vi "GyroServoControl In SbRio.vi"() -> ()   [LabVIEW 2017]
uses:
  MsgTypeDef.ctl
  <vilib>/WPC Systems Ltd/GECO Driver/Lib/GECOMotion/GECOMotion/_typedefine/Axis Select.ctl
  <vilib>/WPC Systems Ltd/GECO Driver/Lib/GECOMotion/GECOMotion/GECO Motion.lvclass
  <vilib>/WPC Systems Ltd/GECO Driver/Lib/GECOBase/GECO_Driver Class/Motion/_typedefine/GECO_ActiveHighLow.ctl
  <vilib>/WPC Systems Ltd/GECO Driver/Lib/GECOBase/GECO_Driver Class/GECO_Driver.lvclass
  <vilib>/WPC Systems Ltd/GECO Driver/Lib/GECOBase/GECO_Driver Class/Motion/_typedefine/GECO_Motion Operation Mode.ctl
  <vilib>/addons/control/pid/NI_PID_pid.lvlib
  <vilib>/addons/control/pid/pid.llb/PID (DBL).vi
  <vilib>/WPC Systems Ltd/GECO Driver/GECODriver/GECO_Initialize_PC/Initialize VIs/Initialize_GECOUno_4HX.vi
  <vilib>/NI/Modbus Library/API/Wrapper/API Main.lvlib
  <vilib>/NI/Modbus Library/API/Wrapper/Create TCP Slave.vi
  <vilib>/NI/Modbus Library/API/Modbus API.lvclass
  <vilib>/Instr/_visa.llb/VISA Configure Serial Port (Instr).vi
  GyroDef.ctl
  <vilib>/WPC Systems Ltd/GECO Driver/Lib/GECOBase/GECO_Driver Class/GECO_SlotName.ctl
  <vilib>/WPC Systems Ltd/GECO Driver/Lib/GECOBase/GECO_Driver Class/Motion/_typedefine/GECO_Stepper Output Configuration.ctl
  DataDef.ctl
  <vilib>/NI/Modbus Library/API/Slave/Modbus Slave.lvclass
  C:/Program Files (x86)/National Instruments/LabVIEW 2019/vi.lib/NI/Modbus Library/API/Modbus API.lvclass
  Reverse Polarity.ctl
  Forward Polarity.ctl
  Motion Controller Slot.ctl
  Stepper Output Configuration.ctl
  Axis Select.ctl
panel:
  out "實際角度":cluster{"X":dbl, "Y":dbl}={"X"=-3.299667554384925, "Y"=3.520332445615068}
  out "實際角度Chart":cluster{"X":dbl, "Y":dbl}(graph)={"X"=-3.299667554384925, "Y"=3.520332445615068} caption="Waveform Chart - dark"
  in  "Main Setting Tab":T1(tab)
  in  "TimerON":bool
  in  "Timer(ms)":i32=1
  in  "Serial Port":refnum<visa-resource-name>="COM3"
  in  "TCP slave port":u32=1
  in  "baud rate":u32=115200
  in  "Byte bits":u32=8
  in  "Modbus Address Starting":u32
  in  "Modbus Number of Inputs":u32=10000
  in  "Resource Name":tag="rio://192.168.0.224/RIO0"
  in  "Servo on":bool
  in  "Axis Select":T2
  in  "Stepper Output Configuration":T3=enum."CW/CCW(Two Pulse)"
  in  "Forward Enable?":bool=TRUE
  in  "Reverse Enable?":bool=TRUE
  in  "Motion Operation Mode":T4(ring)=enum."Velocity"
  in  "Forward Polarity":T5
  in  "Reverse Polarity":T6
  in  "Motion Controller Slot":T7
  in  "Target Position (0)":dbl=10000.0
  in  "Acceleration (100000)":u32=300000
  in  "Velocity (10000)":dbl=100000.0
  in  "Deacceleration (100000)":u32=300000
  in  "PID gains setting Tab":enum32{"Axis 1", "Axis 2", "Axis 3"}(tab)
  in  "PID gains":T8={"proportional gain (Kc)"=1.0, "integral time (Ti, min)"=0.01, "derivative time (Td, min)"=0.0} {"derivative time (Td, min)" format="%#_3f"; "integral time (Ti, min)" format="%#_3f"; "proportional gain (Kc)" format="%#_3f"}
  in  "PID gains 2":T8={"proportional gain (Kc)"=1.0, "integral time (Ti, min)"=0.01, "derivative time (Td, min)"=0.0} {"derivative time (Td, min)" format="%#_3f"; "integral time (Ti, min)" format="%#_3f"; "proportional gain (Kc)" format="%#_3f"}
  in  "PID gains 3":T8={"proportional gain (Kc)"=1.0, "integral time (Ti, min)"=0.01, "derivative time (Td, min)"=0.0} {"derivative time (Td, min)" format="%#_3f"; "integral time (Ti, min)" format="%#_3f"; "proportional gain (Kc)" format="%#_3f"}
  in  "ZABStop":bool
  in  "B":i32
  in  "A":i32
  in  "Z":i32=50
  in  "ZAB Start":bool
  in  "Move Setting":T9
  out "register values":dbl[](array[numeric])
  out "Axis 1":T10
  out "Axis 2":T10
  out "Axis 3":T10
  out "cicrle Period":u32
  out "Program Period":u32
  in  "ServoButtonControl":T11
  in  "Connect":bool
  in  "Close":bool
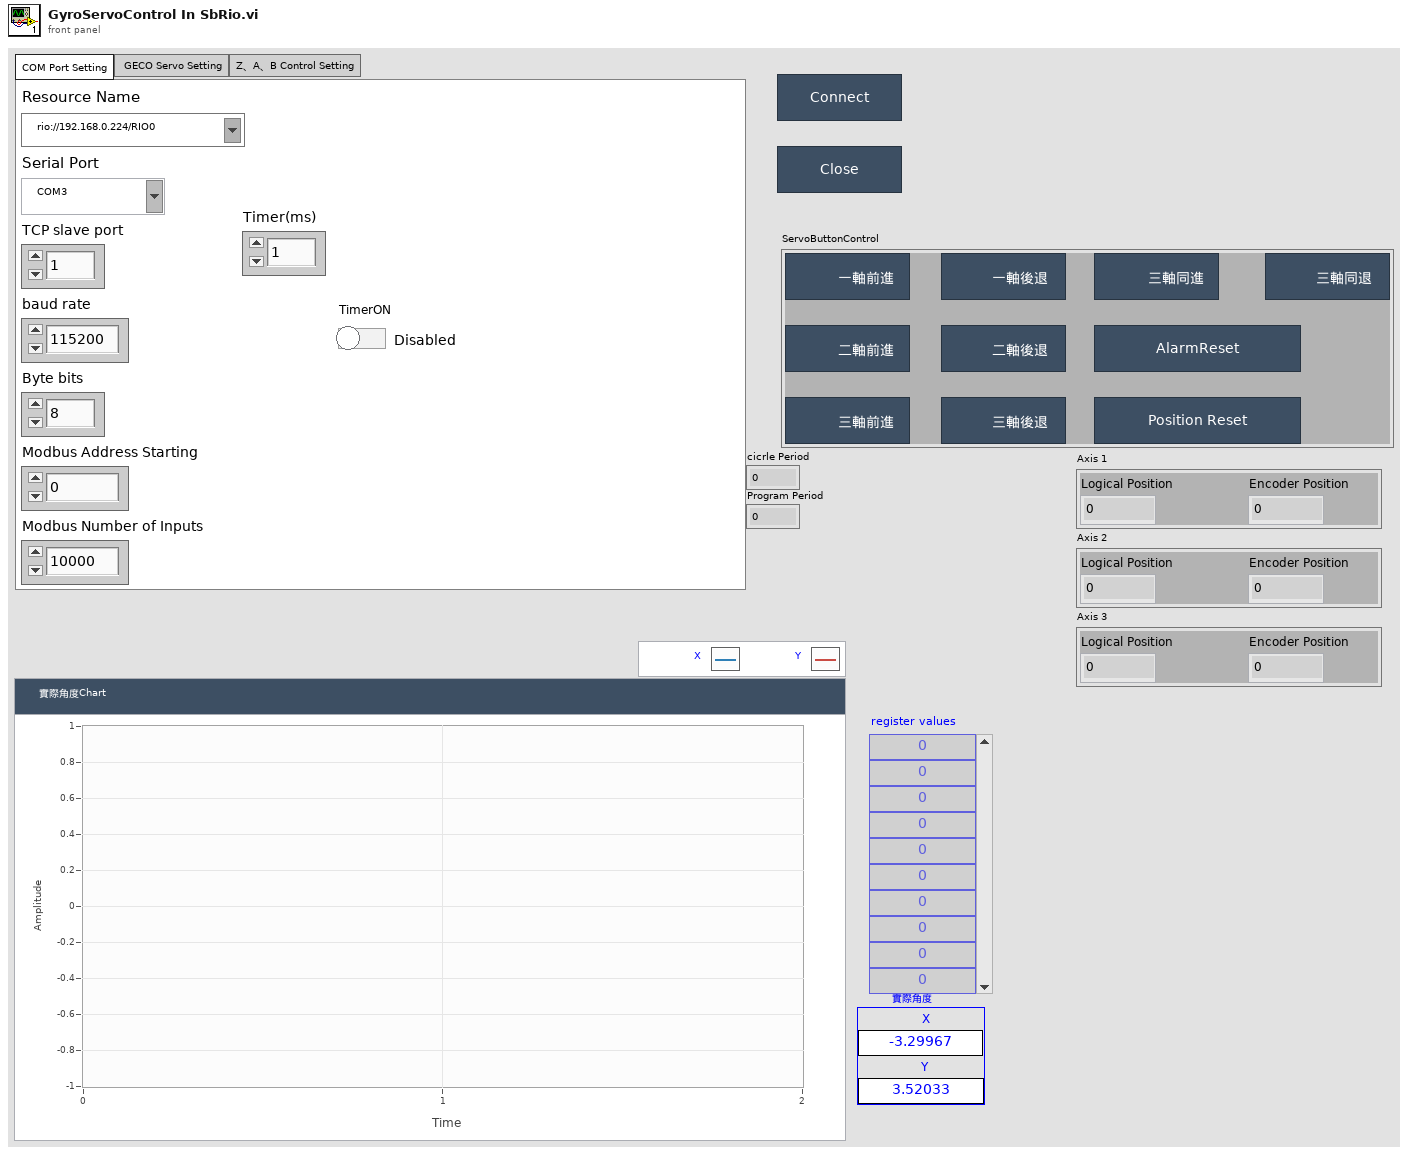
[diagram p1: front panel]
types:
  T1 = enum32{"COM Port Setting", " GECO Servo Setting", "Z、A、B Control Setting"}
  T2 = typedef "Axis Select.ctl" = enum16{"Axis 1", "Axis 2", "Axis 3", "Axis 4"}
  T3 = typedef "Stepper Output Configuration.ctl" = enum16{"Step/Dir(One Pulse)", "CW/CCW(Two Pulse)"}
  T4 = enum16{"Absolute Position", "Relative Position", "Velocity"}
  T5 = typedef "Forward Polarity.ctl" = enum16{"Active High", "Active Low"}
  T6 = typedef "Reverse Polarity.ctl" = enum16{"Active High", "Active Low"}
  T7 = typedef "Motion Controller Slot.ctl" = enum16{"C1", "C2", "C3", "C4"}
  T8 = cluster{"proportional gain (Kc)":dbl, "integral time (Ti, min)":dbl, "derivative time (Td, min)":dbl}
  T9 = typedef "軌跡設定.ctl" = u16
  T10 = cluster{"Encoder Position":i32, "Logical Position":i32}
  T11 = cluster{"三軸同退":bool, "三軸同進":bool, "三軸後退":bool, "三軸前進":bool, "二軸後退":bool, "二軸前進":bool, "一軸後退":bool, "一軸前進":bool, "Reset Encoder Position":bool, "AlarmReset":bool}
  T12 = typedef "DataDef.ctl" = cluster{"address starting":u16, "狀態":enum16{"初始化", "讀取", "寫入", "停止"}, "理想角度":cluster{"A":dbl, "B":dbl}, "register values":i16[], "Modbus COM":refnum<class "Modbus API.lvclass">, "TCP slave port":u16, " baud rate":u32, "Byte bits":u16, "ServoButtonControl":cluster{"三軸同退":bool, "三軸同進":bool, "三軸後退":bool, "三軸前進":bool, "二軸後退":bool, "二軸前進":bool, "一軸後退":bool, "一軸前進":bool}, "Serial Number":string, "GECO_Driver out":refnum<class "GECO_Driver.lvclass">, "number of inputs":u16, "ServoSetting":cluster{"Axis Select":T13, "Stepper Output Configuration":T14, "Motion Operation Mode":T15, "Motion Controller Slot":T16, "Singel Axis Move Paramters":cluster{"Motion Operation Mode":T15, "Target Position (0)":i32, "Velocity (10000)":i32, "Acceleration (100000)":u32, "Deacceleration (100000)":u32}, "Reverse":cluster{"Reverse Enable":bool, "Reverse Polarity":T17}, "Forward":cluster{"Forward Enable":bool, "Forward Polarity":T17}}, "GECO Motion out":refnum<class "GECO Motion.lvclass">, "Servo on":bool, "Axis 1 Position":cluster{"Encoder Position":i32, "Logical Position":i32}, "Axis 2 Position":cluster{"Encoder Position":i32, "Logical Position":i32}, "Axis 3 Position":cluster{"Encoder Position":i32, "Logical Position":i32}, "PIDSetting":cluster{"Z":i32, "A":i32, "B":i32, "Move Setting":T18, "Axis Pulse":dbl, "Axis Length":dbl, "PID gains ":cluster{"proportional gain (Kc)":dbl, "integral time (Ti, min)":dbl, "derivative time (Td, min)":dbl}}, "resource name":tag, "Save Path":refnum<file>}
  T13 = typedef "GECO Motion.lvclass/Axis Select.ctl" = enum16{"Axis 1", "Axis 2", "Axis 3", "Axis 4"}
  T14 = typedef "GECO_Driver.lvclass/GECO_Stepper Output Configuration.ctl" = enum16{"Step/Dir(One Pulse)", "CW/CCW(Two Pulse)"}
  T15 = typedef "GECO_Driver.lvclass/GECO_Motion Operation Mode.ctl" = enum16{"Absolute Position", "Relative Position", "Velocity"}
  T16 = typedef "GECO_Driver.lvclass/GECO_SlotName.ctl" = enum16{"C1", "C2", "C3", "C4"}
  T17 = typedef "GECO_Driver.lvclass/GECO_ActiveHighLow.ctl" = enum16{"Active High", "Active Low"}
  T18 = typedef "­y¸ñ.ctl" = u16
  T19 = typedef "MsgTypeDef.ctl" = cluster{"CMD":string, "DATA":variant}
  T20 = typedef "GyroDef.ctl" = cluster{"Byte bits":u16, "baud rate":u32, "實際角度":cluster{"A":dbl, "B":dbl}, "COM Port":refnum<visa-resource-name>, "Save Path":refnum<file>}
  T21 = cluster{"Motion Operation Mode":T15, "Target Position (0)":i32, "Velocity (10000)":i32, "Acceleration (100000)":u32, "Deacceleration (100000)":u32}
  T22 = cluster{"Forward Enable":bool, "Forward Polarity":T17}
  T23 = cluster{"Reverse Enable":bool, "Reverse Polarity":T17}
  T24 = cluster{"三軸同退":bool, "三軸同進":bool, "三軸後退":bool, "三軸前進":bool, "二軸後退":bool, "二軸前進":bool, "一軸後退":bool, "一軸前進":bool, "Reset Encoder Position":bool, "AlarmReset":bool}[]
  T25 = cluster{"Logical Position":i32, "Encoder Position":i32}
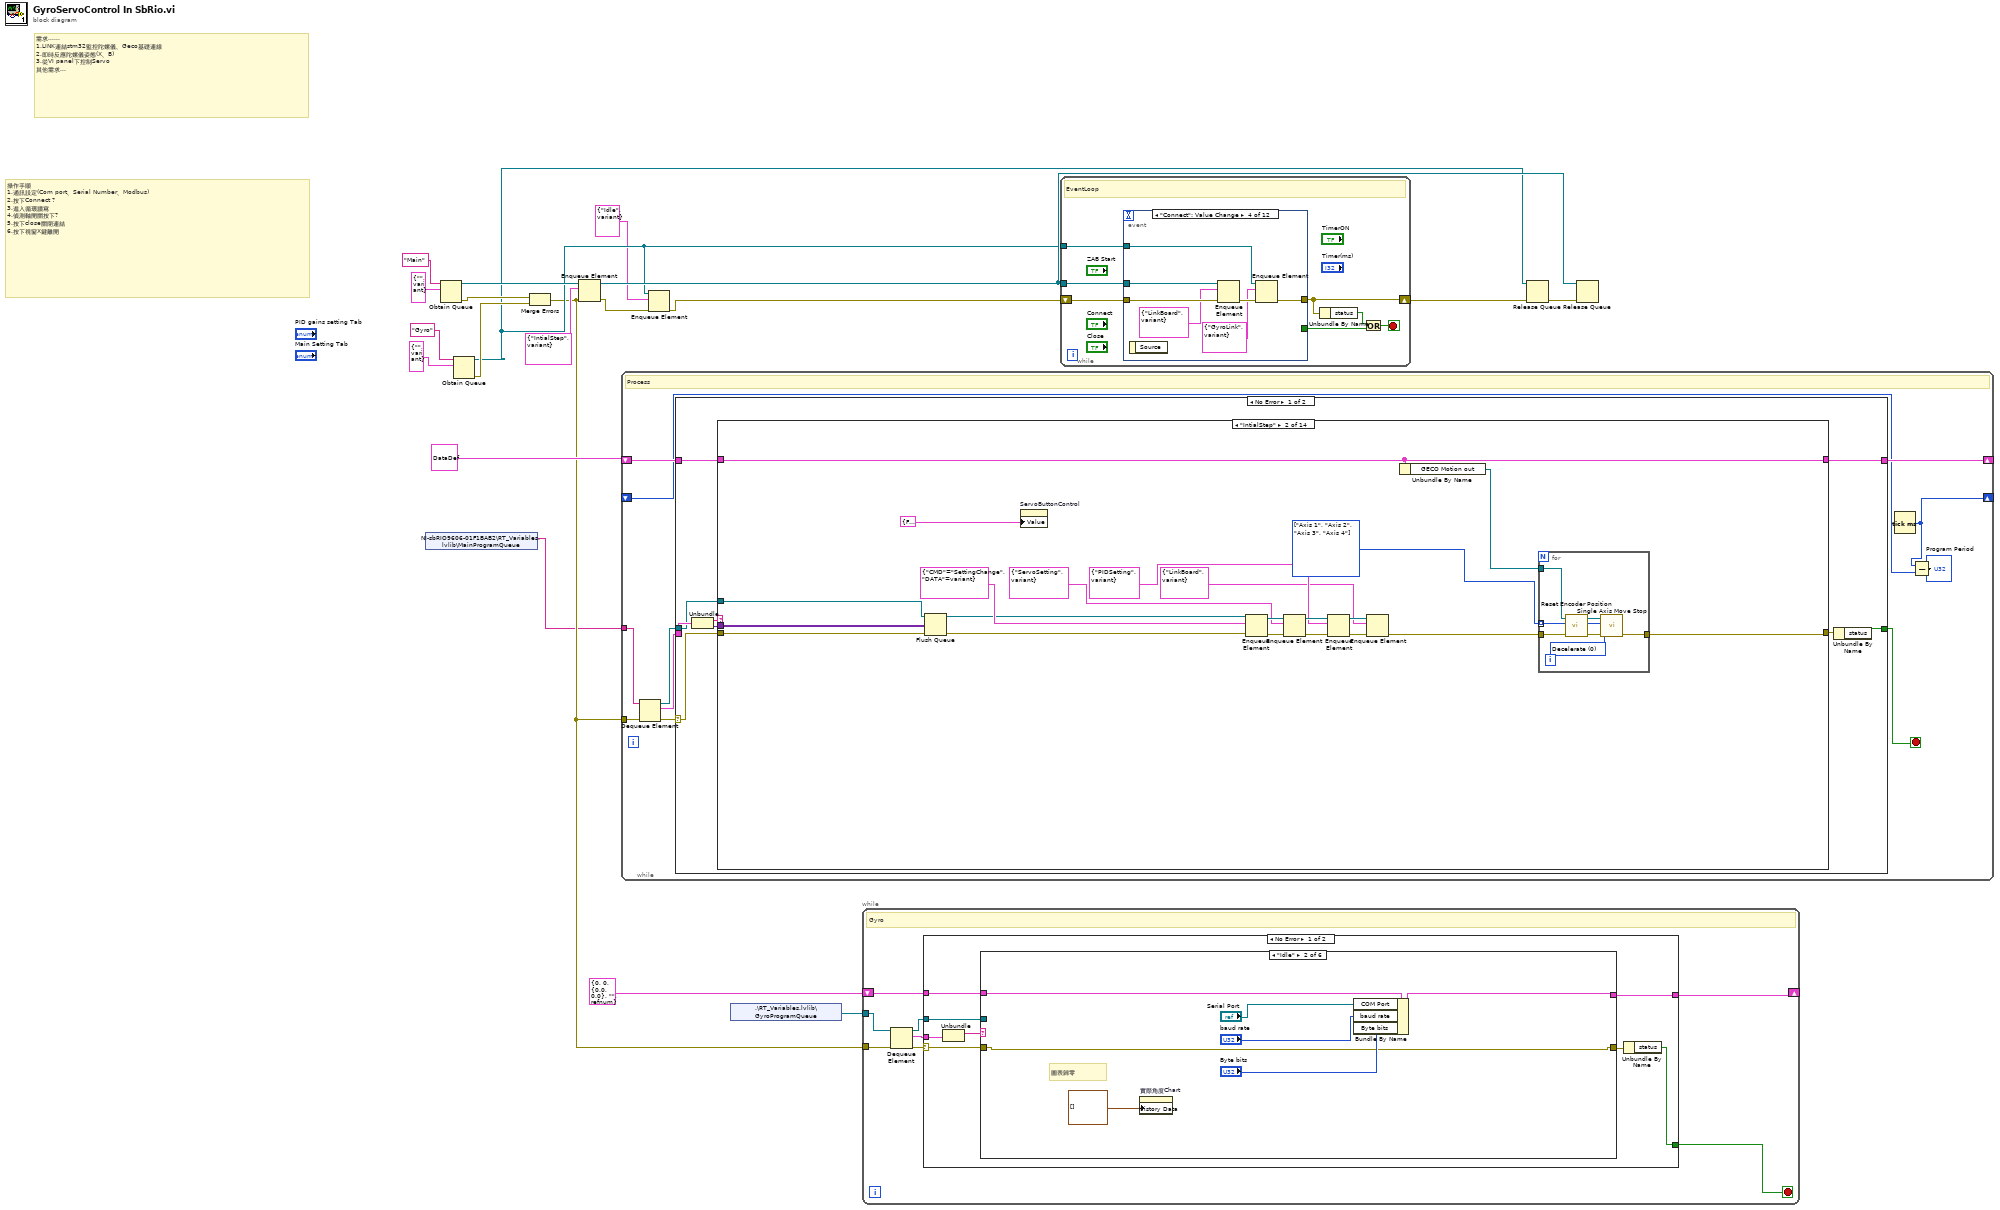
[diagram p0: block diagram]
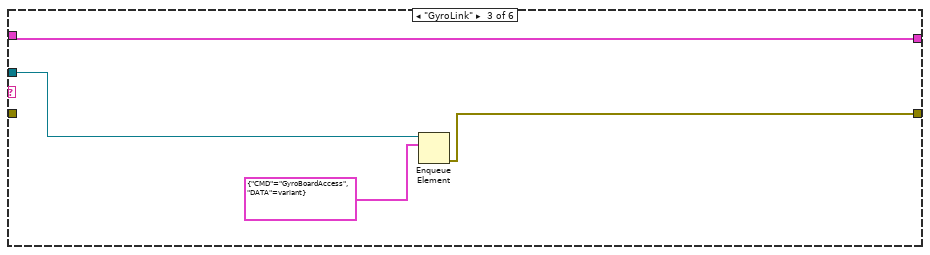
[diagram p3: hidden frame]
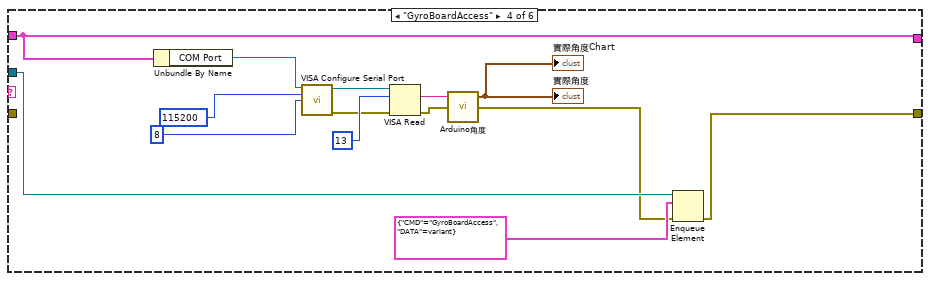
[diagram p4: hidden frame]
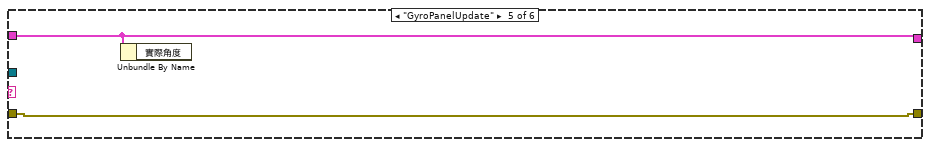
[diagram p5: hidden frame]
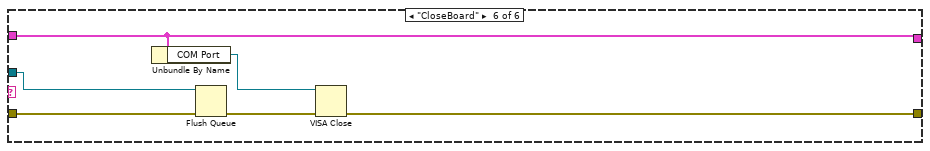
[diagram p6: hidden frame]
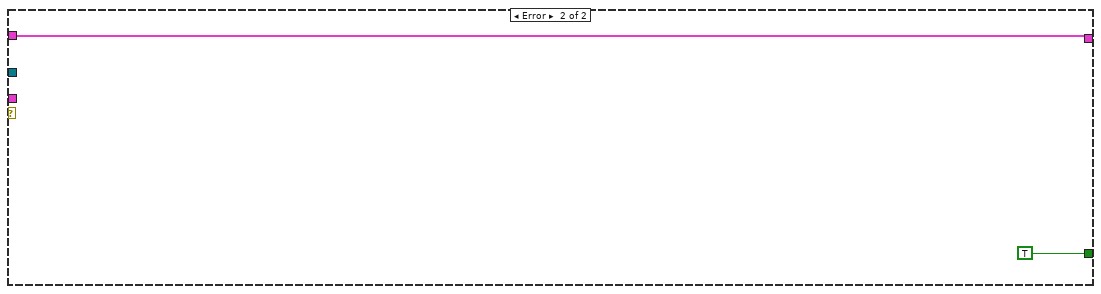
[diagram p7: hidden frame]
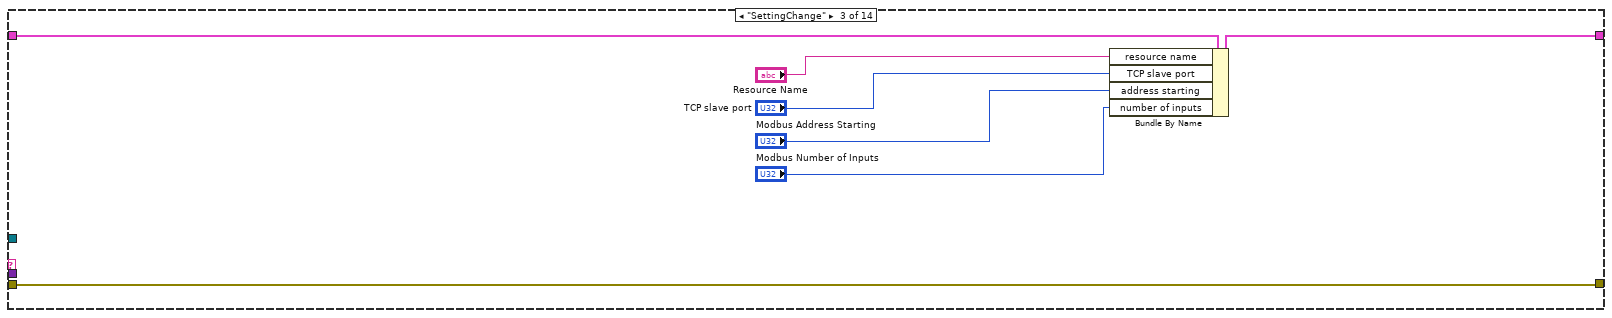
[diagram p9: hidden frame]
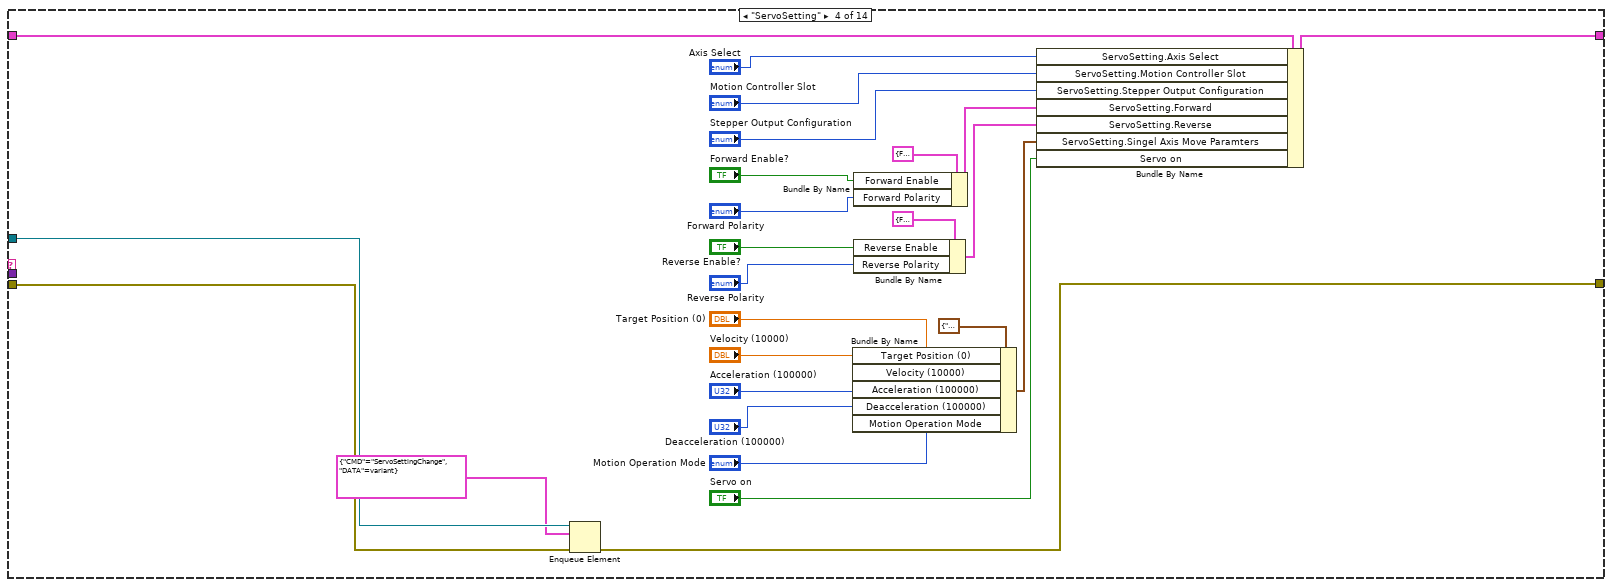
[diagram p10: hidden frame]
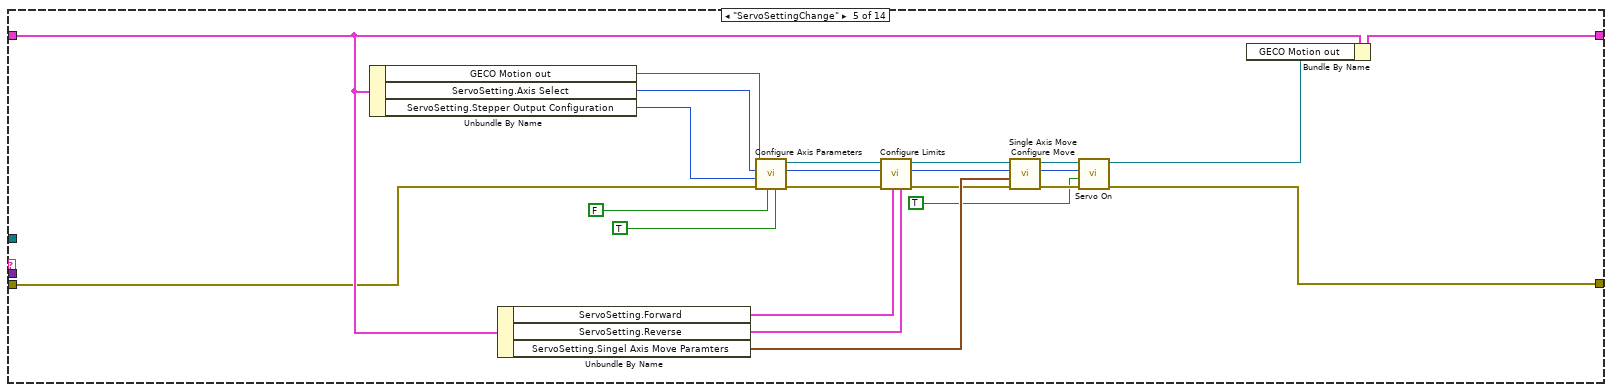
[diagram p11: hidden frame]
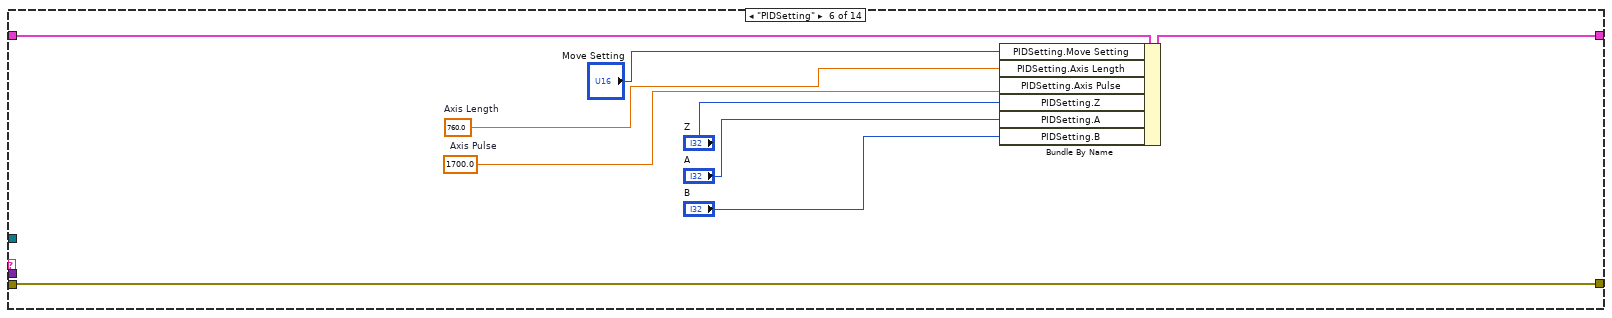
[diagram p12: hidden frame]
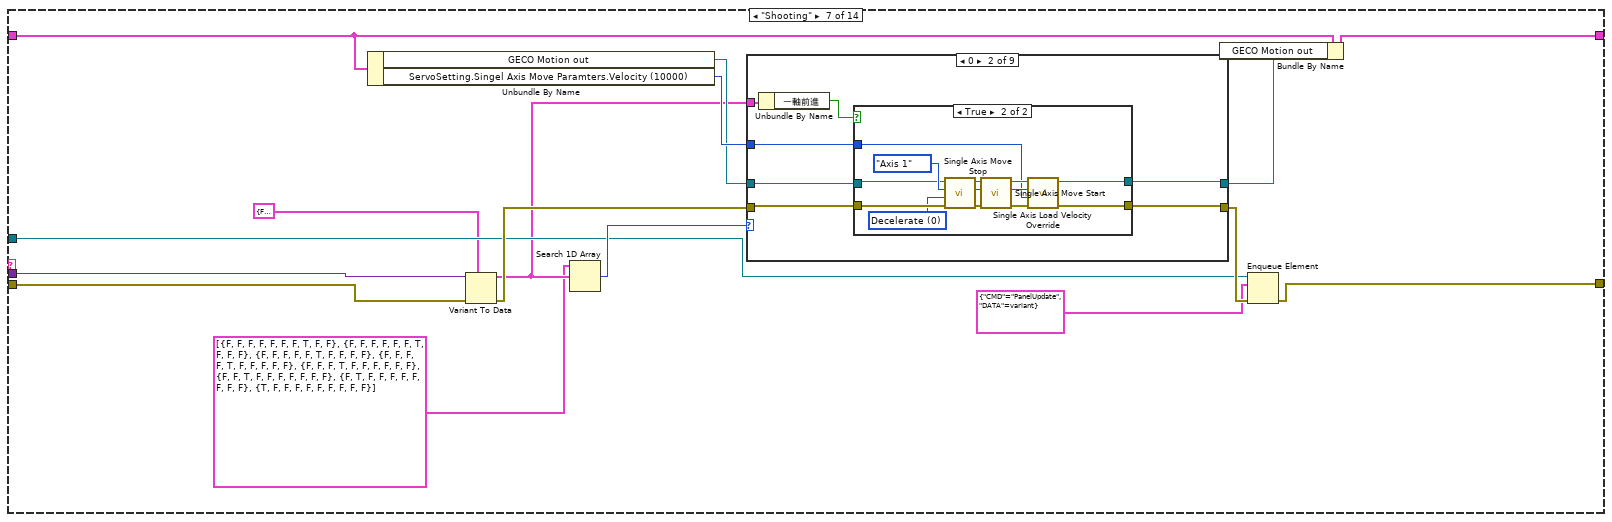
[diagram p13: hidden frame]
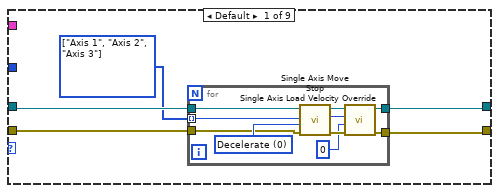
[diagram p14: hidden frame]
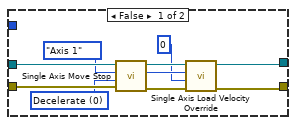
[diagram p15: hidden frame]
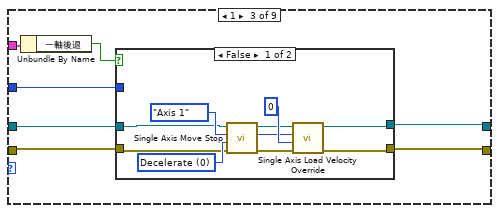
[diagram p16: hidden frame]
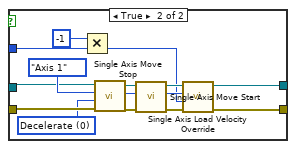
[diagram p17: hidden frame]
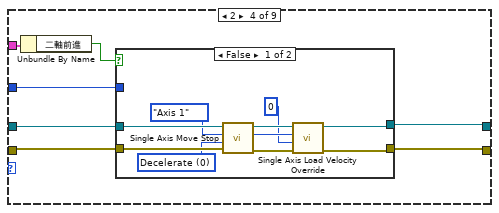
[diagram p18: hidden frame]
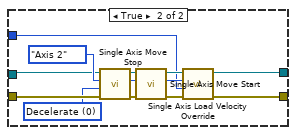
[diagram p19: hidden frame]
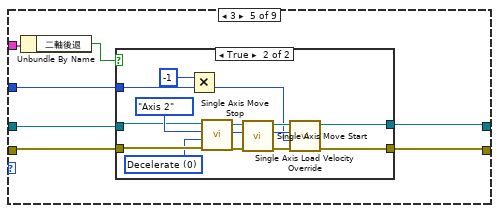
[diagram p20: hidden frame]
diagram:
  # "操作手順\n1.通訊設定(Com port、Serial Number、Modbus)\n2.按下Connect ?\n3.進入循環讀寫\n4.偵測軸開關按下?\n5.按下close關閉連結\n6.按下視窗X鍵離開"
  # "需求......\n1.LINK連結stm32監控陀螺儀、Geco基礎連線\n2.即時反應陀螺儀姿態(X、B)\n3.從VI panel下控制Servo\n其他需求..."
  n1 = shared-variable "NI-sbRIO9606-01F1BAB2\\RT_Variables.lvlib\\MainProgramQueue"() -> (w1:string)  [unwired: 1 in, 1 out]
  n2 = Obtain Queue(name (unnamed)="Main", element data type=T19 {"CMD"="", "DATA"=variant}) -> (queue out=w16:refnum<queue>, error out=w11:errorcluster)  [unwired: 3 in, 1 out]
  n3 = Obtain Queue(name (unnamed)="Gyro", element data type=T19 {"CMD"="", "DATA"=variant}) -> (queue out=w5:refnum<queue>, error out=w12:errorcluster)  [unwired: 3 in, 1 out]
  n4 = Merge Errors(w11, w12) -> (w3:errorcluster)
  n5 = Enqueue Element(queue=w16, element=T19 {"CMD"="IntialStep", "DATA"=variant}, error in (no error)=w3) -> (queue out=w6:refnum<queue>, error out=w8:errorcluster)  [unwired: 1 in, 1 out]
  n6 = while {
    tunnel: w1 -> [w31]
    shift-right: [w27] -> _
    shift-left: T12 {"address starting"=0, "狀態"=enum."初始化", "理想角度"={"A"=0.0, "B"=0.0}, "register values"=[], "Modbus COM"=refnum, "TCP slave port"=1, " baud rate"=0, "Byte bits"=0, "ServoButtonControl"={"三軸同退"=FALSE, "三軸同進"=FALSE, "三軸後退"=FALSE, "三軸前進"=FALSE, "二軸後退"=FALSE, "二軸前進"=FALSE, "一軸後退"=FALSE, "一軸前進"=FALSE}, "Serial Number"="", "GECO_Driver out"=refnum, "number of inputs"=0, "ServoSetting"={"Axis Select"=enum."Axis 1", "Stepper Output Configuration"=enum."Step/Dir(One Pulse)", "Motion Operation Mode"=enum."Absolute Position", "Motion Controller Slot"=enum."C1", "Singel Axis Move Paramters"={"Motion Operation Mode"=enum."Velocity", "Target Position (0)"=10000, "Velocity (10000)"=1, "Acceleration (100000)"=100000, "Deacceleration (100000)"=1}, "Reverse"={"Reverse Enable"=FALSE, "Reverse Polarity"=enum."Active Low"}, "Forward"={"Forward Enable"=FALSE, "Forward Polarity"=enum."Active Low"}}, "GECO Motion out"=refnum, "Servo on"=FALSE, "Axis 1 Position"={"Encoder Position"=0, "Logical Position"=0}, "Axis 2 Position"={"Encoder Position"=0, "Logical Position"=0}, "Axis 3 Position"={"Encoder Position"=0, "Logical Position"=0}, "PIDSetting"={"Z"=10000, "A"=10000, "B"=10000, "Move Setting"=1, "Axis Pulse"=10000.0, "Axis Length"=10000.0, "PID gains "={"proportional gain (Kc)"=1.0, "integral time (Ti, min)"=0.01, "derivative time (Td, min)"=0.0}}, "resource name"="", "Save Path"=refnum} -> [w26]
    tunnel: w3 -> [w24]
    shift-right: [w22] -> _
    shift-left: _ -> [w21]
    stop <- w28 stop-if-true
    # "Process"
    n7 = Dequeue Element(queue=w31, error in (no error)=w24) -> (queue out=w25:refnum<queue>, element=w29:T19, error out=w30:errorcluster)  [unwired: 1 in, 1 out]
    n8 = case shown="No Error" w30 {
      selector: w30 -> [w36 _]
      tunnel: w29 -> [w40 _]
      tunnel: [w32 TRUE] -> w28
      tunnel: [w38 w696] -> w27
      tunnel: w26 -> [w37 w696]
      tunnel: w25 -> [w35 _]
      frame No Error {
        n9 = Unbundle(w40) -> ("CMD"=w39:string, "DATA"=w34:variant)
        n10 = case shown="\"IntialStep\"" w39 {
          tunnel: [w42 w57 w76 w101 w125 w133 w148 w435 w594 w610 w637 w651 w673 w687] -> w38
          tunnel: w37 -> [w42 w57 w77 w102 w124 w134 w142 w437 w597 w613 w638 w652 w675 w687]
          tunnel: w36 -> [w41 w49 w73 w80 w117 w126 w150 w429 w596 w612 w625 w645 w677 w684]
          tunnel: [w41 w56 w73 w78 w111 w126 w139 w436 w592 w608 w634 w642 w676 w686] -> w33
          tunnel: w35 -> [_ w50 _ w81 _ _ w140 w433 _ _ w632 w646 _ w685]
          tunnel: w34 -> [_ _ _ _ _ _ w149 _ _ _ _ _ _ _]
          frame Default {
          }
          frame "IntialStep" {
            w54 = T13[] [enum."Axis 1", enum."Axis 2", enum."Axis 3", enum."Axis 4"] items=["Axis 1", "Axis 2", "Axis 3", "Axis 4"]
            n11 = Flush Queue(queue=w50, error in (no error)=w49) -> (queue out=w48:refnum<queue>, error out=w47:errorcluster)  [unwired: 1 out]
            n12 = property on="ServoButtonControl" class="Clust"("Value"=T11 {"三軸同退"=FALSE, "三軸同進"=FALSE, "三軸後退"=FALSE, "三軸前進"=FALSE, "二軸後退"=FALSE, "二軸前進"=FALSE, "一軸後退"=FALSE, "一軸前進"=FALSE, "Reset Encoder Position"=FALSE, "AlarmReset"=FALSE} ("ServoButtonControl")) -> ()  [unwired: 2 in, 2 out]
            n13 = Enqueue Element(queue=w48, element=T19 {"CMD"="SettingChange", "DATA"=variant}, error in (no error)=w47) -> (queue out=w60:refnum<queue>, error out=w61:errorcluster)  [unwired: 1 in, 1 out]
            n14 = Enqueue Element(queue=w60, element=T19 {"CMD"="ServoSetting", "DATA"=variant}, error in (no error)=w61) -> (queue out=w53:refnum<queue>, error out=w52:errorcluster)  [unwired: 1 in, 1 out]
            n15 = Enqueue Element(queue=w53, element=T19 {"CMD"="PIDSetting", "DATA"=variant}, error in (no error)=w52) -> (queue out=w46:refnum<queue>, error out=w45:errorcluster)  [unwired: 1 in, 1 out]
            n16 = Enqueue Element(queue=w46, element=T19 {"CMD"="LinkBoard", "DATA"=variant}, error in (no error)=w45) -> (error out=w44:errorcluster)  [unwired: 1 in, 2 out]
            n17 = Unbundle By Name(w57) -> ("GECO Motion out"=w55:refnum<class "GECO Motion.lvclass">)
            n18 = for {
              tunnel: w44 -> [w70]
              tunnel: [w64] -> w56
              tunnel: w55 -> [w69]
              tunnel: w54 -> [w68] mode=indexing
              w63 = u16 0 items=["Decelerate", "Halt"] ("Motion Stop Type")
              n19 = call <vilib>:"Reset Encoder Position.vi"("error in (no error)"=w70, "Axis Select"=w68, "GECO Motion in"=w69) -> ("error out"=w67:errorcluster, "Axis Select out"=w66:T13, "GECO Motion out"=w65:refnum<class "GECO Motion.lvclass">)  [unwired: 6 in]
              n20 = call <vilib>:"Single Axis Move Stop.vi"("error in (no error)"=w67, "Motion Stop Type"=w63, "Axis Select"=w66, "GECO Motion in"=w65) -> ("error out"=w64:errorcluster)  [unwired: 5 in, 2 out]
            }
          }
          frame "SettingChange" {
            n21 = Bundle By Name(cluster=w77, "resource name"="Resource Name", "TCP slave port"="TCP slave port", "address starting"="Modbus Address Starting", "number of inputs"="Modbus Number of Inputs") -> (w76:T12)
          }
          frame "ServoSetting" {
            n22 = Enqueue Element(queue=w81, element=T19 {"CMD"="ServoSettingChange", "DATA"=variant}, error in (no error)=w80) -> (error out=w78:errorcluster)  [unwired: 1 in, 2 out]
            n23 = Bundle By Name(cluster=T21 {"Motion Operation Mode"=enum."Absolute Position", "Target Position (0)"=0, "Velocity (10000)"=10000, "Acceleration (100000)"=100000, "Deacceleration (100000)"=100000} ("Singel Axis Move Paramters"), "Target Position (0)"="Target Position (0)", "Velocity (10000)"="Velocity (10000)", "Acceleration (100000)"="Acceleration (100000)", "Deacceleration (100000)"="Deacceleration (100000)", "Motion Operation Mode"="Motion Operation Mode") -> (w83:T21)
            n24 = Bundle By Name(cluster=T22 {"Forward Enable"=FALSE, "Forward Polarity"=enum."Active Low"} ("Forward"), "Forward Enable"="Forward Enable?", "Forward Polarity"="Forward Polarity") -> (w85:T22)
            n25 = Bundle By Name(cluster=T23 {"Reverse Enable"=FALSE, "Reverse Polarity"=enum."Active Low"} ("Reverse"), "Reverse Enable"="Reverse Enable?", "Reverse Polarity"="Reverse Polarity") -> (w84:T23)
            n26 = Bundle By Name(cluster=w102, "ServoSetting.Axis Select"="Axis Select", "ServoSetting.Motion Controller Slot"="Motion Controller Slot", "ServoSetting.Stepper Output Configuration"="Stepper Output Configuration", "ServoSetting.Forward"=w85, "ServoSetting.Reverse"=w84, "ServoSetting.Singel Axis Move Paramters"=w83, "Servo on"="Servo on") -> (w101:T12)
          }
          frame "ServoSettingChange" {
            n27 = Unbundle By Name(w124) -> ("GECO Motion out"=w118:refnum<class "GECO Motion.lvclass">, "ServoSetting.Axis Select"=w122:T13, "ServoSetting.Stepper Output Configuration"=w121:T14)
            n28 = Unbundle By Name(w124) -> ("ServoSetting.Forward"=w104:T22, "ServoSetting.Reverse"=w103:T23, "ServoSetting.Singel Axis Move Paramters"=w123:T21)
            n29 = call <vilib>:"Configure Axis Parameters.vi"("Reverse Encoder Direction?"=TRUE, "Reverse Axis Direction?"=FALSE, "error in (no error)"=w117, "Stepper Output Configuration"=w121, "Axis Select"=w122, "GECO Motion in"=w118) -> ("error out"=w108:errorcluster, "Axis Select out"=w110:T13, "GECO Motion out"=w109:refnum<class "GECO Motion.lvclass">)  [unwired: 3 in]
            n30 = call <vilib>:"Configure Limits.vi"("Reverse"=w103, "Forward"=w104, "error in (no error)"=w108, "Axis Select"=w110, "GECO Motion in"=w109) -> ("error out"=w105:errorcluster, "Axis Select out"=w106:T13, "GECO Motion out"=w107:refnum<class "GECO Motion.lvclass">)  [unwired: 4 in]
            n31 = call <vilib>:"Single Axis Move Configure Move.vi"("error in (no error)"=w105, "Singel Axis Move Paramters"=w123, "Axis Select"=w106, "GECO Motion in"=w107) -> ("error out"=w114:errorcluster, "Axis Select out"=w115:T13, "GECO Motion out"=w116:refnum<class "GECO Motion.lvclass">)  [unwired: 5 in]
            n32 = call <vilib>:"Servo On.vi"("error in (no error)"=w114, "Servo On"=TRUE, "Axis Select"=w115, "GECO Motion in"=w116) -> ("error out"=w111:errorcluster, "GECO Motion out"=w112:refnum<class "GECO Motion.lvclass">)  [unwired: 5 in, 1 out]
            n33 = Bundle By Name(cluster=w124, "GECO Motion out"=w112) -> (w125:T12)
          }
          frame "PIDSetting" {
            w130 = 1700.0  # Axis Pulse
            w131 = 760.0  # Axis Length
            n34 = Bundle By Name(cluster=w134, "PIDSetting.Move Setting"="Move Setting", "PIDSetting.Axis Length"=w131, "PIDSetting.Axis Pulse"=w130, "PIDSetting.Z"="Z", "PIDSetting.A"="A", "PIDSetting.B"="B") -> (w133:T12)
          }
          frame "Shooting" {
            n35 = Unbundle By Name(w142) -> ("GECO Motion out"=w144:refnum<class "GECO Motion.lvclass">, "ServoSetting.Singel Axis Move Paramters.Velocity (10000)"=w145:i32)
            n36 = Variant To Data(error in=w150, type=T11 {"三軸同退"=FALSE, "三軸同進"=FALSE, "三軸後退"=FALSE, "三軸前進"=FALSE, "二軸後退"=FALSE, "二軸前進"=FALSE, "一軸後退"=FALSE, "一軸前進"=FALSE, "Reset Encoder Position"=FALSE, "AlarmReset"=FALSE} ("ServoButtonControl"), Variant=w149) -> (data=w137:T11, error out=w146:errorcluster)
            n37 = Search 1D Array(1D array=T24 [{"三軸同退"=FALSE, "三軸同進"=FALSE, "三軸後退"=FALSE, "三軸前進"=FALSE, "二軸後退"=FALSE, "二軸前進"=FALSE, "一軸後退"=FALSE, "一軸前進"=TRUE, "Reset Encoder Position"=FALSE, "AlarmReset"=FALSE}, {"三軸同退"=FALSE, "三軸同進"=FALSE, "三軸後退"=FALSE, "三軸前進"=FALSE, "二軸後退"=FALSE, "二軸前進"=FALSE, "一軸後退"=TRUE, "一軸前進"=FALSE, "Reset Encoder Position"=FALSE, "AlarmReset"=FALSE}, {"三軸同退"=FALSE, "三軸同進"=FALSE, "三軸後退"=FALSE, "三軸前進"=FALSE, "二軸後退"=FALSE, "二軸前進"=TRUE, "一軸後退"=FALSE, "一軸前進"=FALSE, "Reset Encoder Position"=FALSE, "AlarmReset"=FALSE}, {"三軸同退"=FALSE, "三軸同進"=FALSE, "三軸後退"=FALSE, "三軸前進"=FALSE, "二軸後退"=TRUE, "二軸前進"=FALSE, "一軸後退"=FALSE, "一軸前進"=FALSE, "Reset Encoder Position"=FALSE, "AlarmReset"=FALSE}, {"三軸同退"=FALSE, "三軸同進"=FALSE, "三軸後退"=FALSE, "三軸前進"=TRUE, "二軸後退"=FALSE, "二軸前進"=FALSE, "一軸後退"=FALSE, "一軸前進"=FALSE, "Reset Encoder Position"=FALSE, "AlarmReset"=FALSE}, {"三軸同退"=FALSE, "三軸同進"=FALSE, "三軸後退"=TRUE, "三軸前進"=FALSE, "二軸後退"=FALSE, "二軸前進"=FALSE, "一軸後退"=FALSE, "一軸前進"=FALSE, "Reset Encoder Position"=FALSE, "AlarmReset"=FALSE}, {"三軸同退"=FALSE, "三軸同進"=TRUE, "三軸後退"=FALSE, "三軸前進"=FALSE, "二軸後退"=FALSE, "二軸前進"=FALSE, "一軸後退"=FALSE, "一軸前進"=FALSE, "Reset Encoder Position"=FALSE, "AlarmReset"=FALSE}, {"三軸同退"=TRUE, "三軸同進"=FALSE, "三軸後退"=FALSE, "三軸前進"=FALSE, "二軸後退"=FALSE, "二軸前進"=FALSE, "一軸後退"=FALSE, "一軸前進"=FALSE, "Reset Encoder Position"=FALSE, "AlarmReset"=FALSE}], element=w137) -> (index of element=w147:i32)  [unwired: 1 in]
            n38 = case shown="0" w147 {
              tunnel: w146 -> [w154 w171 w201 w233 w263 w295 w325 w357 w394]
              tunnel: w145 -> [_ w170 w200 w232 w262 w294 w324 w356 w393]
              tunnel: w144 -> [w155 w172 w202 w234 w264 w296 w326 w358 w395]
              tunnel: [w152 w169 w199 w231 w261 w293 w323 w355 w392] -> w143
              tunnel: [w151 w168 w198 w230 w260 w292 w322 w354 w391] -> w141
              tunnel: w137 -> [_ w167 w197 w229 w259 w291 w321 w353 w390]
              frame Default {
                w153 = T13[] [enum."Axis 1", enum."Axis 2", enum."Axis 3"] items=["Axis 1", "Axis 2", "Axis 3", "Axis 4"] ("Start Axes Select")
                n39 = for {
                  tunnel: w154 -> [w164]
                  tunnel: w155 -> [w163]
                  tunnel: w153 -> [w162] mode=indexing
                  tunnel: [w157] -> w152
                  tunnel: [w158] -> w151
                  w165 = u16 0 items=["Decelerate", "Halt"] ("Motion Stop Type")
                  n40 = call <vilib>:"Single Axis Move Stop.vi"("error in (no error)"=w164, "Motion Stop Type"=w165, "Axis Select"=w162, "GECO Motion in"=w163) -> ("error out"=w160:errorcluster, "Axis Select out"=w159:T13, "GECO Motion out"=w161:refnum<class "GECO Motion.lvclass">)  [unwired: 5 in]
                  n41 = call <vilib>:"Single Axis Load Velocity Override.vi"("error in (no error)"=w160, "Override Velosity Value"=0, "Axis Select"=w159, "GECO Motion in"=w161) -> ("error out"=w158:errorcluster, "GECO Motion out"=w157:refnum<class "GECO Motion.lvclass">)  [unwired: 5 in, 1 out]
                }
              }
              frame 0 {
                n42 = Unbundle By Name(w167) -> ("一軸前進"=w166:bool)
                n43 = case shown="True" w166 {
                  tunnel: w172 -> [w182 w188]
                  tunnel: w171 -> [w181 w187]
                  tunnel: w170 -> [_ w192]
                  tunnel: [w173 w191] -> w169
                  tunnel: [w174 w190] -> w168
                  frame False {
                    w180 = u16 0 items=["Decelerate", "Halt"] ("Motion Stop Type")
                    n44 = call <vilib>:"Single Axis Move Stop.vi"("error in (no error)"=w181, "Motion Stop Type"=w180, "Axis Select"=Axis_Select."Axis 1", "GECO Motion in"=w182) -> ("error out"=w177:errorcluster, "Axis Select out"=w176:T13, "GECO Motion out"=w178:refnum<class "GECO Motion.lvclass">)  [unwired: 5 in]
                    n45 = call <vilib>:"Single Axis Load Velocity Override.vi"("error in (no error)"=w177, "Override Velosity Value"=0, "Axis Select"=w176, "GECO Motion in"=w178) -> ("error out"=w174:errorcluster, "GECO Motion out"=w173:refnum<class "GECO Motion.lvclass">)  [unwired: 5 in, 1 out]
                  }
                  frame True {
                    w186 = u16 0 items=["Decelerate", "Halt"] ("Motion Stop Type")
                    n46 = call <vilib>:"Single Axis Move Stop.vi"("error in (no error)"=w187, "Motion Stop Type"=w186, "Axis Select"=Axis_Select."Axis 1", "GECO Motion in"=w188) -> ("error out"=w184:errorcluster, "Axis Select out"=w183:T13, "GECO Motion out"=w185:refnum<class "GECO Motion.lvclass">)  [unwired: 5 in]
                    n47 = call <vilib>:"Single Axis Move Start.vi"("error in (no error)"=w184, "Axis Select"=w183, "GECO Motion in"=w185) -> ("error out"=w194:errorcluster, "Axis Select out"=w193:T13, "GECO Motion out"=w195:refnum<class "GECO Motion.lvclass">)  [unwired: 6 in]
                    n48 = call <vilib>:"Single Axis Load Velocity Override.vi"("error in (no error)"=w194, "Override Velosity Value"=w192, "Axis Select"=w193, "GECO Motion in"=w195) -> ("error out"=w190:errorcluster, "GECO Motion out"=w191:refnum<class "GECO Motion.lvclass">)  [unwired: 5 in, 1 out]
                  }
                }
              }
              frame 1 {
                n49 = Unbundle By Name(w197) -> ("一軸後退"=w196:bool)
                n50 = case shown="False" w196 {
                  tunnel: w202 -> [w208 w216]
                  tunnel: w201 -> [w206 w215]
                  tunnel: w200 -> [_ w224]
                  tunnel: [w210 w223] -> w199
                  tunnel: [w211 w222] -> w198
                  frame False {
                    w207 = u16 0 items=["Decelerate", "Halt"] ("Motion Stop Type")
                    n51 = call <vilib>:"Single Axis Move Stop.vi"("error in (no error)"=w206, "Motion Stop Type"=w207, "Axis Select"=Axis_Select."Axis 1", "GECO Motion in"=w208) -> ("error out"=w204:errorcluster, "Axis Select out"=w203:T13, "GECO Motion out"=w205:refnum<class "GECO Motion.lvclass">)  [unwired: 5 in]
                    n52 = call <vilib>:"Single Axis Load Velocity Override.vi"("error in (no error)"=w204, "Override Velosity Value"=0, "Axis Select"=w203, "GECO Motion in"=w205) -> ("error out"=w211:errorcluster, "GECO Motion out"=w210:refnum<class "GECO Motion.lvclass">)  [unwired: 5 in, 1 out]
                  }
                  frame True {
                    w214 = u16 0 items=["Decelerate", "Halt"] ("Motion Stop Type")
                    n53 = Multiply(x=-1, y=w224) -> (x*y=w221:i32)
                    n54 = call <vilib>:"Single Axis Move Stop.vi"("error in (no error)"=w215, "Motion Stop Type"=w214, "Axis Select"=Axis_Select."Axis 1", "GECO Motion in"=w216) -> ("error out"=w218:errorcluster, "Axis Select out"=w213:T13, "GECO Motion out"=w219:refnum<class "GECO Motion.lvclass">)  [unwired: 5 in]
                    n55 = call <vilib>:"Single Axis Move Start.vi"("error in (no error)"=w218, "Axis Select"=w213, "GECO Motion in"=w219) -> ("error out"=w226:errorcluster, "Axis Select out"=w225:T13, "GECO Motion out"=w227:refnum<class "GECO Motion.lvclass">)  [unwired: 6 in]
                    n56 = call <vilib>:"Single Axis Load Velocity Override.vi"("error in (no error)"=w226, "Override Velosity Value"=w221, "Axis Select"=w225, "GECO Motion in"=w227) -> ("error out"=w222:errorcluster, "GECO Motion out"=w223:refnum<class "GECO Motion.lvclass">)  [unwired: 5 in, 1 out]
                  }
                }
              }
              frame 2 {
                n57 = Unbundle By Name(w229) -> ("二軸前進"=w228:bool)
                n58 = case shown="False" w228 {
                  tunnel: w234 -> [w244 w250]
                  tunnel: w233 -> [w243 w249]
                  tunnel: w232 -> [_ w254]
                  tunnel: [w235 w253] -> w231
                  tunnel: [w236 w252] -> w230
                  frame False {
                    w242 = u16 0 items=["Decelerate", "Halt"] ("Motion Stop Type")
                    n59 = call <vilib>:"Single Axis Move Stop.vi"("error in (no error)"=w243, "Motion Stop Type"=w242, "Axis Select"=Axis_Select."Axis 1", "GECO Motion in"=w244) -> ("error out"=w239:errorcluster, "Axis Select out"=w238:T13, "GECO Motion out"=w240:refnum<class "GECO Motion.lvclass">)  [unwired: 5 in]
                    n60 = call <vilib>:"Single Axis Load Velocity Override.vi"("error in (no error)"=w239, "Override Velosity Value"=0, "Axis Select"=w238, "GECO Motion in"=w240) -> ("error out"=w236:errorcluster, "GECO Motion out"=w235:refnum<class "GECO Motion.lvclass">)  [unwired: 5 in, 1 out]
                  }
                  frame True {
                    w248 = u16 0 items=["Decelerate", "Halt"] ("Motion Stop Type")
                    n61 = call <vilib>:"Single Axis Move Stop.vi"("error in (no error)"=w249, "Motion Stop Type"=w248, "Axis Select"=Axis_Select."Axis 2", "GECO Motion in"=w250) -> ("error out"=w246:errorcluster, "Axis Select out"=w245:T13, "GECO Motion out"=w247:refnum<class "GECO Motion.lvclass">)  [unwired: 5 in]
                    n62 = call <vilib>:"Single Axis Move Start.vi"("error in (no error)"=w246, "Axis Select"=w245, "GECO Motion in"=w247) -> ("error out"=w256:errorcluster, "Axis Select out"=w255:T13, "GECO Motion out"=w257:refnum<class "GECO Motion.lvclass">)  [unwired: 6 in]
                    n63 = call <vilib>:"Single Axis Load Velocity Override.vi"("error in (no error)"=w256, "Override Velosity Value"=w254, "Axis Select"=w255, "GECO Motion in"=w257) -> ("error out"=w252:errorcluster, "GECO Motion out"=w253:refnum<class "GECO Motion.lvclass">)  [unwired: 5 in, 1 out]
                  }
                }
              }
              frame 3 {
                n64 = Unbundle By Name(w259) -> ("二軸後退"=w258:bool)
                n65 = case shown="True" w258 {
                  tunnel: w264 -> [w274 w278]
                  tunnel: w263 -> [w273 w277]
                  tunnel: w262 -> [_ w286]
                  tunnel: [w265 w285] -> w261
                  tunnel: [w266 w284] -> w260
                  frame False {
                    w272 = u16 0 items=["Decelerate", "Halt"] ("Motion Stop Type")
                    n66 = call <vilib>:"Single Axis Move Stop.vi"("error in (no error)"=w273, "Motion Stop Type"=w272, "Axis Select"=Axis_Select."Axis 1", "GECO Motion in"=w274) -> ("error out"=w269:errorcluster, "Axis Select out"=w268:T13, "GECO Motion out"=w270:refnum<class "GECO Motion.lvclass">)  [unwired: 5 in]
                    n67 = call <vilib>:"Single Axis Load Velocity Override.vi"("error in (no error)"=w269, "Override Velosity Value"=0, "Axis Select"=w268, "GECO Motion in"=w270) -> ("error out"=w266:errorcluster, "GECO Motion out"=w265:refnum<class "GECO Motion.lvclass">)  [unwired: 5 in, 1 out]
                  }
                  frame True {
                    w276 = u16 0 items=["Decelerate", "Halt"] ("Motion Stop Type")
                    n68 = Multiply(x=-1, y=w286) -> (x*y=w283:i32)
                    n69 = call <vilib>:"Single Axis Move Stop.vi"("error in (no error)"=w277, "Motion Stop Type"=w276, "Axis Select"=Axis_Select."Axis 2", "GECO Motion in"=w278) -> ("error out"=w280:errorcluster, "Axis Select out"=w275:T13, "GECO Motion out"=w281:refnum<class "GECO Motion.lvclass">)  [unwired: 5 in]
                    n70 = call <vilib>:"Single Axis Move Start.vi"("error in (no error)"=w280, "Axis Select"=w275, "GECO Motion in"=w281) -> ("error out"=w288:errorcluster, "Axis Select out"=w287:T13, "GECO Motion out"=w289:refnum<class "GECO Motion.lvclass">)  [unwired: 6 in]
                    n71 = call <vilib>:"Single Axis Load Velocity Override.vi"("error in (no error)"=w288, "Override Velosity Value"=w283, "Axis Select"=w287, "GECO Motion in"=w289) -> ("error out"=w284:errorcluster, "GECO Motion out"=w285:refnum<class "GECO Motion.lvclass">)  [unwired: 5 in, 1 out]
                  }
                }
              }
              frame 4 {
                n72 = Unbundle By Name(w291) -> ("三軸前進"=w290:bool)
                n73 = case shown="False" w290 {
                  tunnel: w296 -> [w306 w312]
                  tunnel: w295 -> [w305 w311]
                  tunnel: w294 -> [_ w316]
                  tunnel: [w297 w315] -> w293
                  tunnel: [w298 w314] -> w292
                  frame False {
                    w304 = u16 0 items=["Decelerate", "Halt"] ("Motion Stop Type")
                    n74 = call <vilib>:"Single Axis Move Stop.vi"("error in (no error)"=w305, "Motion Stop Type"=w304, "Axis Select"=Axis_Select."Axis 1", "GECO Motion in"=w306) -> ("error out"=w301:errorcluster, "Axis Select out"=w300:T13, "GECO Motion out"=w302:refnum<class "GECO Motion.lvclass">)  [unwired: 5 in]
                    n75 = call <vilib>:"Single Axis Load Velocity Override.vi"("error in (no error)"=w301, "Override Velosity Value"=0, "Axis Select"=w300, "GECO Motion in"=w302) -> ("error out"=w298:errorcluster, "GECO Motion out"=w297:refnum<class "GECO Motion.lvclass">)  [unwired: 5 in, 1 out]
                  }
                  frame True {
                    w310 = u16 0 items=["Decelerate", "Halt"] ("Motion Stop Type")
                    n76 = call <vilib>:"Single Axis Move Stop.vi"("error in (no error)"=w311, "Motion Stop Type"=w310, "Axis Select"=Axis_Select."Axis 3", "GECO Motion in"=w312) -> ("error out"=w308:errorcluster, "Axis Select out"=w307:T13, "GECO Motion out"=w309:refnum<class "GECO Motion.lvclass">)  [unwired: 5 in]
                    n77 = call <vilib>:"Single Axis Move Start.vi"("error in (no error)"=w308, "Axis Select"=w307, "GECO Motion in"=w309) -> ("error out"=w318:errorcluster, "Axis Select out"=w317:T13, "GECO Motion out"=w319:refnum<class "GECO Motion.lvclass">)  [unwired: 6 in]
                    n78 = call <vilib>:"Single Axis Load Velocity Override.vi"("error in (no error)"=w318, "Override Velosity Value"=w316, "Axis Select"=w317, "GECO Motion in"=w319) -> ("error out"=w314:errorcluster, "GECO Motion out"=w315:refnum<class "GECO Motion.lvclass">)  [unwired: 5 in, 1 out]
                  }
                }
              }
              frame 5 {
                n79 = Unbundle By Name(w321) -> ("三軸後退"=w320:bool)
                n80 = case shown="False" w320 {
                  tunnel: w326 -> [w336 w340]
                  tunnel: w325 -> [w335 w339]
                  tunnel: w324 -> [_ w348]
                  tunnel: [w327 w347] -> w323
                  tunnel: [w328 w346] -> w322
                  frame False {
                    w334 = u16 0 items=["Decelerate", "Halt"] ("Motion Stop Type")
                    n81 = call <vilib>:"Single Axis Move Stop.vi"("error in (no error)"=w335, "Motion Stop Type"=w334, "Axis Select"=Axis_Select."Axis 1", "GECO Motion in"=w336) -> ("error out"=w331:errorcluster, "Axis Select out"=w330:T13, "GECO Motion out"=w332:refnum<class "GECO Motion.lvclass">)  [unwired: 5 in]
                    n82 = call <vilib>:"Single Axis Load Velocity Override.vi"("error in (no error)"=w331, "Override Velosity Value"=0, "Axis Select"=w330, "GECO Motion in"=w332) -> ("error out"=w328:errorcluster, "GECO Motion out"=w327:refnum<class "GECO Motion.lvclass">)  [unwired: 5 in, 1 out]
                  }
                  frame True {
                    w338 = u16 0 items=["Decelerate", "Halt"] ("Motion Stop Type")
                    n83 = Multiply(x=-1, y=w348) -> (x*y=w345:i32)
                    n84 = call <vilib>:"Single Axis Move Stop.vi"("error in (no error)"=w339, "Motion Stop Type"=w338, "Axis Select"=Axis_Select."Axis 3", "GECO Motion in"=w340) -> ("error out"=w342:errorcluster, "Axis Select out"=w337:T13, "GECO Motion out"=w343:refnum<class "GECO Motion.lvclass">)  [unwired: 5 in]
                    n85 = call <vilib>:"Single Axis Move Start.vi"("error in (no error)"=w342, "Axis Select"=w337, "GECO Motion in"=w343) -> ("error out"=w350:errorcluster, "Axis Select out"=w349:T13, "GECO Motion out"=w351:refnum<class "GECO Motion.lvclass">)  [unwired: 6 in]
                    n86 = call <vilib>:"Single Axis Load Velocity Override.vi"("error in (no error)"=w350, "Override Velosity Value"=w345, "Axis Select"=w349, "GECO Motion in"=w351) -> ("error out"=w346:errorcluster, "GECO Motion out"=w347:refnum<class "GECO Motion.lvclass">)  [unwired: 5 in, 1 out]
                  }
                }
              }
              frame 6 {
                n87 = Unbundle By Name(w353) -> ("三軸同進"=w352:bool)
                n88 = case shown="False" w352 {
                  tunnel: w358 -> [w362 w380]
                  tunnel: w357 -> [w363 w379]
                  tunnel: w356 -> [_ w375]
                  tunnel: [w360 w388] -> w355
                  tunnel: [w359 w387] -> w354
                  frame False {
                    w361 = T13[] [enum."Axis 1", enum."Axis 2", enum."Axis 3"] items=["Axis 1", "Axis 2", "Axis 3", "Axis 4"] ("Start Axes Select")
                    n89 = for {
                      tunnel: w363 -> [w372]
                      tunnel: w362 -> [w371]
                      tunnel: w361 -> [w370] mode=indexing
                      tunnel: [w365] -> w360
                      tunnel: [w366] -> w359
                      w373 = u16 0 items=["Decelerate", "Halt"] ("Motion Stop Type")
                      n90 = call <vilib>:"Single Axis Move Stop.vi"("error in (no error)"=w372, "Motion Stop Type"=w373, "Axis Select"=w370, "GECO Motion in"=w371) -> ("error out"=w368:errorcluster, "Axis Select out"=w367:T13, "GECO Motion out"=w369:refnum<class "GECO Motion.lvclass">)  [unwired: 5 in]
                      n91 = call <vilib>:"Single Axis Load Velocity Override.vi"("error in (no error)"=w368, "Override Velosity Value"=0, "Axis Select"=w367, "GECO Motion in"=w369) -> ("error out"=w366:errorcluster, "GECO Motion out"=w365:refnum<class "GECO Motion.lvclass">)  [unwired: 5 in, 1 out]
                    }
                  }
                  frame True {
                    w376 = T13[] [enum."Axis 1", enum."Axis 2", enum."Axis 3"] items=["Axis 1", "Axis 2", "Axis 3", "Axis 4"] ("Start Axes Select")
                    n92 = call <vilib>:"Single Axis Load Velocity Override.vi"("error in (no error)"=w379, "Override Velosity Value"=w375, "Axis Select"=Axis_Select."Axis 1", "GECO Motion in"=w380) -> ("error out"=w385:errorcluster, "GECO Motion out"=w386:refnum<class "GECO Motion.lvclass">)  [unwired: 5 in, 1 out]
                    n93 = call <vilib>:"Single Axis Load Velocity Override.vi"("error in (no error)"=w385, "Override Velosity Value"=w375, "Axis Select"=Axis_Select."Axis 2", "GECO Motion in"=w386) -> ("error out"=w383:errorcluster, "GECO Motion out"=w384:refnum<class "GECO Motion.lvclass">)  [unwired: 5 in, 1 out]
                    n94 = call <vilib>:"Single Axis Load Velocity Override.vi"("error in (no error)"=w383, "Override Velosity Value"=w375, "Axis Select"=Axis_Select."Axis 3", "GECO Motion in"=w384) -> ("error out"=w381:errorcluster, "GECO Motion out"=w382:refnum<class "GECO Motion.lvclass">)  [unwired: 5 in, 1 out]
                    n95 = call <vilib>:"MultiAxes Sync Move Start.vi"("error in (no error)"=w381, "Start Axes Select"=w376, "GECO Motion in"=w382) -> ("error out"=w387:errorcluster, "GECO Motion out"=w388:refnum<class "GECO Motion.lvclass">)  [unwired: 7 in]
                  }
                }
              }
              frame 7 {
                n96 = Unbundle By Name(w390) -> ("三軸同退"=w389:bool)
                n97 = case shown="False" w389 {
                  tunnel: w395 -> [w399 w419]
                  tunnel: w394 -> [w400 w418]
                  tunnel: w393 -> [_ w412]
                  tunnel: [w397 w427] -> w392
                  tunnel: [w396 w426] -> w391
                  frame False {
                    w398 = T13[] [enum."Axis 1", enum."Axis 2", enum."Axis 3"] items=["Axis 1", "Axis 2", "Axis 3", "Axis 4"] ("Start Axes Select")
                    n98 = for {
                      tunnel: w400 -> [w409]
                      tunnel: w399 -> [w408]
                      tunnel: w398 -> [w407] mode=indexing
                      tunnel: [w402] -> w397
                      tunnel: [w403] -> w396
                      w410 = u16 0 items=["Decelerate", "Halt"] ("Motion Stop Type")
                      n99 = call <vilib>:"Single Axis Move Stop.vi"("error in (no error)"=w409, "Motion Stop Type"=w410, "Axis Select"=w407, "GECO Motion in"=w408) -> ("error out"=w405:errorcluster, "Axis Select out"=w404:T13, "GECO Motion out"=w406:refnum<class "GECO Motion.lvclass">)  [unwired: 5 in]
                      n100 = call <vilib>:"Single Axis Load Velocity Override.vi"("error in (no error)"=w405, "Override Velosity Value"=0, "Axis Select"=w404, "GECO Motion in"=w406) -> ("error out"=w403:errorcluster, "GECO Motion out"=w402:refnum<class "GECO Motion.lvclass">)  [unwired: 5 in, 1 out]
                    }
                  }
                  frame True {
                    w415 = T13[] [enum."Axis 1", enum."Axis 2", enum."Axis 3"] items=["Axis 1", "Axis 2", "Axis 3", "Axis 4"] ("Start Axes Select")
                    n101 = Multiply(x=w412, y=-1) -> (x*y=w413:i32)
                    n102 = call <vilib>:"Single Axis Load Velocity Override.vi"("error in (no error)"=w418, "Override Velosity Value"=w413, "Axis Select"=Axis_Select."Axis 1", "GECO Motion in"=w419) -> ("error out"=w424:errorcluster, "GECO Motion out"=w425:refnum<class "GECO Motion.lvclass">)  [unwired: 5 in, 1 out]
                    n103 = call <vilib>:"Single Axis Load Velocity Override.vi"("error in (no error)"=w424, "Override Velosity Value"=w413, "Axis Select"=Axis_Select."Axis 2", "GECO Motion in"=w425) -> ("error out"=w422:errorcluster, "GECO Motion out"=w423:refnum<class "GECO Motion.lvclass">)  [unwired: 5 in, 1 out]
                    n104 = call <vilib>:"Single Axis Load Velocity Override.vi"("error in (no error)"=w422, "Override Velosity Value"=w413, "Axis Select"=Axis_Select."Axis 3", "GECO Motion in"=w423) -> ("error out"=w420:errorcluster, "GECO Motion out"=w421:refnum<class "GECO Motion.lvclass">)  [unwired: 5 in, 1 out]
                    n105 = call <vilib>:"MultiAxes Sync Move Start.vi"("error in (no error)"=w420, "Start Axes Select"=w415, "GECO Motion in"=w421) -> ("error out"=w426:errorcluster, "GECO Motion out"=w427:refnum<class "GECO Motion.lvclass">)  [unwired: 7 in]
                  }
                }
              }
            }
            n106 = Bundle By Name(cluster=w142, "GECO Motion out"=w143) -> (w148:T12)
            n107 = Enqueue Element(queue=w140, element=T19 {"CMD"="PanelUpdate", "DATA"=variant}, error in (no error)=w141) -> (error out=w139:errorcluster)  [unwired: 1 in, 2 out]
          }
          frame "ZABMove" {
            n108 = Unbundle By Name(w437) -> ("PIDSetting.Move Setting"=w438:T18, "GECO Motion out"=w428:refnum<class "GECO Motion.lvclass">)
            n109 = case shown="1" w438 {
              selector: w438 -> [_ w458 w512 _ _]
              tunnel: w437 -> [_ w480 w504 w588 w591]
              tunnel: w429 -> [w443 w489 w506 w587 w590]
              tunnel: [w442 w450 w507 w587 w590] -> w436
              tunnel: [w441 w459 w511 w586 w589] -> w434
              tunnel: w433 -> [_ w452 w502 _ _]
              tunnel: [_ _ w510 _ _] -> w432
              tunnel: [_ _ w509 _ _] -> w431
              tunnel: [_ _ w508 _ _] -> w430
              tunnel: w428 -> [w439 _ w505 _ _]
              frame Default {
                w440 = T13[] [enum."Axis 1", enum."Axis 2", enum."Axis 3", enum."Axis 4"] items=["Axis 1", "Axis 2", "Axis 3", "Axis 4"]
                n110 = for {
                  tunnel: w443 -> [w446]
                  tunnel: [w444] -> w442
                  tunnel: [w445] -> w441
                  tunnel: w440 -> [w448] mode=indexing
                  tunnel: w439 -> [w449]
                  w447 = u16 0 items=["Decelerate", "Halt"] ("Motion Stop Type")
                  n111 = call <vilib>:"Single Axis Move Stop.vi"("error in (no error)"=w446, "Motion Stop Type"=w447, "Axis Select"=w448, "GECO Motion in"=w449) -> ("error out"=w444:errorcluster, "GECO Motion out"=w445:refnum<class "GECO Motion.lvclass">)  [unwired: 5 in, 1 out]
                }
              }
              frame 0 {
                w468 = T13[] [enum."Axis 1", enum."Axis 2", enum."Axis 3"] items=["Axis 1", "Axis 2", "Axis 3", "Axis 4"] ("Start Axes Select")
                # "輸入Z、A、B"
                n112 = Unbundle By Name(w480) -> ("PIDSetting.Z"=w486:i32, "PIDSetting.A"=w485:i32, "PIDSetting.B"=w484:i32, "PIDSetting.Axis Length"=w494:dbl, "PIDSetting.Axis Pulse"=w490:dbl, "GECO Motion out"=w488:refnum<class "GECO Motion.lvclass">)
                n113 = Unbundle By Name(w480) -> ("ServoSetting.Singel Axis Move Paramters.Velocity (10000)"=w463:i32)
                n114 = call "綜合圓軌跡子VI.vi"("Ring"=w458, "移動z"=w486, "al"=w485, "be"=w484) -> ("Z"=w460:dbl, "A"=w461:dbl, "B"=w462:dbl)  [unwired: 2 in]
                n115 = call "推導公式.vi"("be"=w462, "al"=w461, "移動z"=w460) -> ("L3"=w495:dbl, "L2"=w496:dbl, "L1"=w497:dbl)
                n116 = Subtract(x=w497, y=w494) -> (x-y=w493:dbl)
                n117 = Subtract(x=w496, y=w494) -> (x-y=w492:dbl)
                n118 = Subtract(x=w495, y=w494) -> (x-y=w491:dbl)
                n119 = Multiply(x=w493, y=w490) -> (x*y=w456:dbl)
                n120 = Multiply(x=w492, y=w490) -> (x*y=w465:dbl)
                n121 = Multiply(x=w491, y=w490) -> (x*y=w457:dbl)
                n122 = call <vilib>:"Single Axis Load Velocity Override.vi"("error in (no error)"=w489, "Override Velosity Value"=w463, "Axis Select"=Axis_Select."Axis 1" ("Single Axis Select"), "GECO Motion in"=w488) -> ("error out"=w482:errorcluster, "Axis Select out"=w481:T13, "GECO Motion out"=w483:refnum<class "GECO Motion.lvclass">)  [unwired: 5 in]
                n123 = call <vilib>:"Single Axis Load Position Override.vi"("error in (no error)"=w482, "Override Target Position Value"=w457, "Axis Select"=w481, "GECO Motion in"=w483) -> ("error out"=w478:errorcluster, "GECO Motion out"=w479:refnum<class "GECO Motion.lvclass">)  [unwired: 5 in, 1 out]
                n124 = call <vilib>:"Single Axis Load Velocity Override.vi"("error in (no error)"=w478, "Override Velosity Value"=w463, "Axis Select"=Axis_Select."Axis 2" ("Single Axis Select"), "GECO Motion in"=w479) -> ("error out"=w475:errorcluster, "Axis Select out"=w474:T13, "GECO Motion out"=w476:refnum<class "GECO Motion.lvclass">)  [unwired: 5 in]
                n125 = call <vilib>:"Single Axis Load Position Override.vi"("error in (no error)"=w475, "Override Target Position Value"=w465, "Axis Select"=w474, "GECO Motion in"=w476) -> ("error out"=w469:errorcluster, "GECO Motion out"=w470:refnum<class "GECO Motion.lvclass">)  [unwired: 5 in, 1 out]
                n126 = call <vilib>:"Single Axis Load Velocity Override.vi"("error in (no error)"=w469, "Override Velosity Value"=w463, "Axis Select"=Axis_Select."Axis 3" ("Single Axis Select"), "GECO Motion in"=w470) -> ("error out"=w472:errorcluster, "Axis Select out"=w471:T13, "GECO Motion out"=w473:refnum<class "GECO Motion.lvclass">)  [unwired: 5 in]
                n127 = call <vilib>:"Single Axis Load Position Override.vi"("error in (no error)"=w472, "Override Target Position Value"=w456, "Axis Select"=w471, "GECO Motion in"=w473) -> ("error out"=w466:errorcluster, "GECO Motion out"=w467:refnum<class "GECO Motion.lvclass">)  [unwired: 5 in, 1 out]
                n128 = call <vilib>:"MultiAxes Sync Move Start.vi"("error in (no error)"=w466, "Start Axes Select"=w468, "GECO Motion in"=w467) -> ("error out"=w451:errorcluster, "GECO Motion out"=w459:refnum<class "GECO Motion.lvclass">)  [unwired: 7 in]
                n129 = Flush Queue(queue=w452, error in (no error)=w451) -> (queue out=w455:refnum<queue>, error out=w454:errorcluster)  [unwired: 1 out]
                n130 = Enqueue Element(queue=w455, element=T19 {"CMD"="BoardAccess", "DATA"=variant}, error in (no error)=w454) -> (error out=w450:errorcluster)  [unwired: 1 in, 2 out]
              }
              frame 1 {
                w498 = 0 ("Encoder Position")
                # "圓軌跡"
                n131 = while {
                  tunnel: w512 -> [w585]
                  tunnel: [w584] -> w510
                  tunnel: [w583] -> w509
                  tunnel: [w582] -> w508
                  tunnel: w504 -> [w538]
                  tunnel: w506 -> [w528]
                  tunnel: [w523] -> w503
                  tunnel: w505 -> [w529]
                  tunnel: [w524] -> w511
                  shift-right: [w535] -> _
                  shift-left: w498 -> [w532]
                  shift-right: [w534] -> _
                  shift-left: w498 -> [w531]
                  shift-right: [w533] -> _
                  shift-left: w498 -> [w530]
                  shift-right: [w522] -> _
                  shift-left: _ -> [w521]
                  i -> [w536]
                  stop <- "ZABStop" stop-if-true
                  w513 = 50000
                  w525 = T13[] [enum."Axis 1", enum."Axis 2", enum."Axis 3"] items=["Axis 1", "Axis 2", "Axis 3", "Axis 4"] ("Start Axes Select")
                  w581 = cluster{"output high":dbl, "output low":dbl} {"output high"=300000.0, "output low"=-300000.0} ("PID Def Output range")
                  w546 = Axis_Select."Axis 3" ("Single Axis Select")
                  w547 = Axis_Select."Axis 2" ("Single Axis Select")
                  w545 = Axis_Select."Axis 1" ("Single Axis Select")
                  # "PID取樣時間"
                  # "Stm32 Delay Time"
                  n132 = Unbundle By Name(w538) -> ("PIDSetting.Axis Length"=w554:dbl, "PIDSetting.Axis Pulse"=w571:dbl)
                  n133 = call <vilib>:"Read Encoder Position.vi"("error in (no error)"=w528, "Axis Select"=w545, "GECO Motion in"=w529) -> ("error out"=w552:errorcluster, "GECO Motion out"=w553:refnum<class "GECO Motion.lvclass">, "Encoder Position"=w535:i32, "Logical Position"=w542:i32)  [unwired: 4 in, 1 out]
                  n134 = call <vilib>:"Read Encoder Position.vi"("error in (no error)"=w552, "Axis Select"=w547, "GECO Motion in"=w553) -> ("error out"=w550:errorcluster, "GECO Motion out"=w551:refnum<class "GECO Motion.lvclass">, "Encoder Position"=w534:i32, "Logical Position"=w541:i32)  [unwired: 4 in, 1 out]
                  n135 = Bundle("Encoder Position"=w535, "Logical Position"=w542) -> (w584:T10)  [unwired: 1 in]
                  n136 = call <vilib>:"Read Encoder Position.vi"("error in (no error)"=w550, "Axis Select"=w546, "GECO Motion in"=w551) -> ("error out"=w548:errorcluster, "GECO Motion out"=w549:refnum<class "GECO Motion.lvclass">, "Encoder Position"=w533:i32, "Logical Position"=w540:i32)  [unwired: 4 in, 1 out]
                  n137 = call "綜合圓軌跡子VI.vi"("Ring"=w585, "I時間"=w536) -> ("Z"=w578:dbl, "A"=w543:dbl, "B"=w544:dbl)  [unwired: 4 in]
                  n138 = property on="Axis 1" class="Clust (strict)"("Value"=w584) -> ()  [unwired: 2 in, 2 out]
                  n139 = call "推導公式.vi"("be"=w544, "al"=w543, "移動z"=w578) -> ("L3"=w572:dbl, "L2"=w573:dbl, "L1"=w574:dbl)
                  n140 = Bundle("Encoder Position"=w534, "Logical Position"=w541) -> (w583:T10)  [unwired: 1 in]
                  n141 = Subtract(x=w574, y=w554) -> (x-y=w577:dbl)
                  n142 = Subtract(x=w573, y=w554) -> (x-y=w576:dbl)
                  n143 = Subtract(x=w572, y=w554) -> (x-y=w575:dbl)
                  n144 = Divide(x=30.0, y=1000.0) -> (x/y=w567:dbl)
                  n145 = property on="Axis 2" class="Clust (strict)"("Value"=w583) -> ()  [unwired: 2 in, 2 out]
                  n146 = Multiply ("L1 pulse")(x=w577, y=w571) -> (x*y=w517:dbl)
                  n147 = Multiply ("L2 pulse")(x=w576, y=w571) -> (x*y=w518:dbl)
                  n148 = Multiply ("L3 pulse")(x=w575, y=w571) -> (x*y=w519:dbl)
                  n149 = Bundle("Encoder Position"=w533, "Logical Position"=w540) -> (w582:T10)  [unwired: 1 in]
                  n150 = property on="Axis 3" class="Clust (strict)"("Value"=w582) -> ()  [unwired: 2 in, 2 out]
                  n151 = call-poly <vilib>:"PID.vi"("output range"=w581, "dt (s)"=w567, "PID gains"="PID gains", "process variable"=w532, "setpoint"=w519) -> ("output"=w516:dbl)  [unwired: 5 in, 1 out]
                  n152 = call-poly <vilib>:"PID.vi"("output range"=w581, "dt (s)"=w567, "PID gains"="PID gains 2", "process variable"=w531, "setpoint"=w518) -> ("output"=w515:dbl)  [unwired: 5 in, 1 out]
                  n153 = call-poly <vilib>:"PID.vi"("output range"=w581, "dt (s)"=w567, "PID gains"="PID gains 3", "process variable"=w530, "setpoint"=w517) -> ("output"=w514:dbl)  [unwired: 5 in, 1 out]
                  n154 = call <vilib>:"Single Axis Load Velocity Override.vi"("error in (no error)"=w548, "Override Velosity Value"=w513, "Axis Select"=w545, "GECO Motion in"=w549) -> ("error out"=w565:errorcluster, "Axis Select out"=w557:T13, "GECO Motion out"=w566:refnum<class "GECO Motion.lvclass">)  [unwired: 5 in]
                  n155 = call <vilib>:"Single Axis Load Position Override.vi"("error in (no error)"=w565, "Override Target Position Value"=w516, "Axis Select"=w557, "GECO Motion in"=w566) -> ("error out"=w563:errorcluster, "GECO Motion out"=w564:refnum<class "GECO Motion.lvclass">)  [unwired: 5 in, 1 out]
                  n156 = call <vilib>:"Single Axis Load Velocity Override.vi"("error in (no error)"=w563, "Override Velosity Value"=w513, "Axis Select"=w547, "GECO Motion in"=w564) -> ("error out"=w539:errorcluster, "Axis Select out"=w556:T13, "GECO Motion out"=w562:refnum<class "GECO Motion.lvclass">)  [unwired: 5 in]
                  n157 = call <vilib>:"Single Axis Load Position Override.vi"("error in (no error)"=w539, "Override Target Position Value"=w515, "Axis Select"=w556, "GECO Motion in"=w562) -> ("error out"=w560:errorcluster, "GECO Motion out"=w561:refnum<class "GECO Motion.lvclass">)  [unwired: 5 in, 1 out]
                  n158 = call <vilib>:"Single Axis Load Velocity Override.vi"("error in (no error)"=w560, "Override Velosity Value"=w513, "Axis Select"=w546, "GECO Motion in"=w561) -> ("error out"=w558:errorcluster, "Axis Select out"=w555:T13, "GECO Motion out"=w559:refnum<class "GECO Motion.lvclass">)  [unwired: 5 in]
                  n159 = call <vilib>:"Single Axis Load Position Override.vi"("error in (no error)"=w558, "Override Target Position Value"=w514, "Axis Select"=w555, "GECO Motion in"=w559) -> ("error out"=w526:errorcluster, "GECO Motion out"=w527:refnum<class "GECO Motion.lvclass">)  [unwired: 5 in, 1 out]
                  n160 = Tick Count (ms)() -> (millisecond timer value=w522:u32)
                  n161 = Subtract(x=w522, y=w521) -> (x-y=→"cicrle Period":u32)
                  n162 = call <vilib>:"MultiAxes Sync Move Start.vi"("error in (no error)"=w526, "Start Axes Select"=w525, "GECO Motion in"=w527) -> ("error out"=w523:errorcluster, "GECO Motion out"=w524:refnum<class "GECO Motion.lvclass">)  [unwired: 7 in]
                }
                n163 = Flush Queue(queue=w502, error in (no error)=w503) -> (queue out=w501:refnum<queue>, error out=w500:errorcluster)  [unwired: 1 out]
                n164 = Enqueue Element(queue=w501, element=T19 {"CMD"="BoardAccess", "DATA"=variant}, error in (no error)=w500) -> (error out=w507:errorcluster)  [unwired: 1 in, 2 out]
              }
              frame 2 {
                # "Á³±Û­y¸ñ"
                n165 = Unbundle By Name(w588) -> ("GECO Motion out"=w586:refnum<class "GECO Motion.lvclass">)
              }
              frame 3 {
                # "Z上下"
                n166 = Unbundle By Name(w591) -> ("GECO Motion out"=w589:refnum<class "GECO Motion.lvclass">)
              }
            }
            n167 = Bundle By Name(cluster=w437, "GECO Motion out"=w434, "Axis 1 Position"=w432, "Axis 2 Position"=w431, "Axis 3 Position"=w430) -> (w435:T12)
          }
          frame "AlarmReset" {
            w598 = T13[] [enum."Axis 1", enum."Axis 2", enum."Axis 3", enum."Axis 4"] items=["Axis 1", "Axis 2", "Axis 3", "Axis 4"]
            n168 = Unbundle By Name(w597) -> ("GECO Motion out"=w595:refnum<class "GECO Motion.lvclass">)
            n169 = for {
              tunnel: [w607] -> w593
              tunnel: [w606] -> w592
              tunnel: w598 -> [w601] mode=indexing
              tunnel: w596 -> [w603]
              tunnel: w595 -> [w602]
              w599 = u16 0 items=["Decelerate", "Halt"] ("Motion Stop Type")
              n170 = call <vilib>:"Single Axis Move Stop.vi"("error in (no error)"=w603, "Motion Stop Type"=w599, "Axis Select"=w601, "GECO Motion in"=w602) -> ("error out"=w604:errorcluster, "Axis Select out"=w600:T13, "GECO Motion out"=w605:refnum<class "GECO Motion.lvclass">)  [unwired: 5 in]
              n171 = call <vilib>:"Alarm Reset.vi"("error in (no error)"=w604, "Axis Select"=w600, "GECO Motion in"=w605) -> ("error out"=w606:errorcluster, "GECO Motion out"=w607:refnum<class "GECO Motion.lvclass">)  [unwired: 6 in, 1 out]
            }
            n172 = Bundle By Name(cluster=w597, "GECO Motion out"=w593) -> (w594:T12)
          }
          frame "EncoderReset" {
            w614 = T13[] [enum."Axis 1", enum."Axis 2", enum."Axis 3", enum."Axis 4"] items=["Axis 1", "Axis 2", "Axis 3", "Axis 4"]
            n173 = Unbundle By Name(w613) -> ("GECO Motion out"=w611:refnum<class "GECO Motion.lvclass">)
            n174 = for {
              tunnel: [w623] -> w609
              tunnel: [w622] -> w608
              tunnel: w614 -> [w621] mode=indexing
              tunnel: w612 -> [w618]
              tunnel: w611 -> [w617]
              w615 = u16 0 items=["Decelerate", "Halt"] ("Motion Stop Type")
              n175 = call <vilib>:"Single Axis Move Stop.vi"("error in (no error)"=w618, "Motion Stop Type"=w615, "Axis Select"=w621, "GECO Motion in"=w617) -> ("error out"=w619:errorcluster, "Axis Select out"=w616:T13, "GECO Motion out"=w620:refnum<class "GECO Motion.lvclass">)  [unwired: 5 in]
              n176 = call <vilib>:"Reset Encoder Position.vi"("error in (no error)"=w619, "Axis Select"=w616, "GECO Motion in"=w620) -> ("error out"=w622:errorcluster, "GECO Motion out"=w623:refnum<class "GECO Motion.lvclass">)  [unwired: 6 in, 1 out]
            }
            n177 = Bundle By Name(cluster=w613, "GECO Motion out"=w609) -> (w610:T12)
          }
          frame "LinkBoard" {
            n178 = Unbundle By Name(w638) -> ("resource name"=w624:tag, "TCP slave port"=w636:u16, "ServoSetting.Motion Controller Slot"=w626:T16)
            n179 = call-poly <vilib>:"Create Modbus Instance.vi"("error in"=w625, "port (502)"=w636) -> ("error out"=w635:errorcluster, "TCP slave instance"=w627:refnum<class "Modbus Slave.lvclass">)  [unwired: 8 in]
            n180 = call-poly <vilib>:"Initialize.vi"("error in (no error)"=w635, "resource name"=w624) -> ("error out"=w631:errorcluster, "GECO_Driver out"=w628:refnum<class "GECO_Driver.lvclass">)  [unwired: 8 in]
            n181 = call <vilib>:"Initialize Motion Controller.vi"("error in (no error)"=w631, "Slot"=w626, "GECO_Driver in"=w628) -> ("error out"=w629:errorcluster, "Motion reference out"=w630:refnum<class "GECO Motion.lvclass">)  [unwired: 7 in]
            n182 = Bundle By Name(cluster=w638, "Modbus COM"=w627, "GECO_Driver out"=w628, "GECO Motion out"=w630) -> (w637:T12)
            n183 = Enqueue Element(queue=w632, element=T19 {"CMD"="BoardAccess", "DATA"=variant}, error in (no error)=w629) -> (error out=w634:errorcluster)  [unwired: 1 in, 2 out]
          }
          frame "BoardAccess" {
            n184 = Unbundle By Name(w652) -> ("Modbus COM"=w649:refnum<class "Modbus API.lvclass">, "address starting"=w648:u16, "number of inputs"=w647:u16)
            n185 = call-dynamic "Read Holding Registers.vi"("error in"=w645, "number of inputs"=w647, "starting address"=w648, "Modbus instance in"=w649) -> ("error out"=w639:errorcluster, "register values"=w650:u16[])  [unwired: 5 in, 1 out]
            n186 = Enqueue Element(queue=w646, element=T19 {"CMD"="PanelUpdate", "DATA"=variant}, error in (no error)=w639) -> (queue out=w644:refnum<queue>, error out=w643:errorcluster)  [unwired: 1 in, 1 out]
            n187 = Bundle By Name(cluster=w652, "register values"=w650) -> (w651:T12)
            n188 = Enqueue Element(queue=w644, element=T19 {"CMD"="BoardAccess", "DATA"=variant}, error in (no error)=w643) -> (error out=w642:errorcluster)  [unwired: 1 in, 2 out]
          }
          frame "PanelUpdate" {
            n189 = Unbundle By Name(w675) -> ("GECO Motion out"=w674:refnum<class "GECO Motion.lvclass">)
            n190 = call <vilib>:"Read Encoder Position.vi"("error in (no error)"=w677, "Axis Select"=Axis_Select."Axis 1", "GECO Motion in"=w674) -> ("error out"=w670:errorcluster, "GECO Motion out"=w671:refnum<class "GECO Motion.lvclass">, "Encoder Position"=w663:i32, "Logical Position"=w664:i32)  [unwired: 4 in, 1 out]
            n191 = Bundle(cluster=T25 {"Logical Position"=0, "Encoder Position"=0} ("input cluster"), "Logical Position"=w664, "Encoder Position"=w663) -> (w655:T25)
            "Axis 1" <- w655
            n192 = call <vilib>:"Read Encoder Position.vi"("error in (no error)"=w670, "Axis Select"=Axis_Select."Axis 2", "GECO Motion in"=w671) -> ("error out"=w668:errorcluster, "GECO Motion out"=w669:refnum<class "GECO Motion.lvclass">, "Encoder Position"=w656:i32, "Logical Position"=w657:i32)  [unwired: 4 in, 1 out]
            n193 = Bundle(cluster=T25 {"Logical Position"=0, "Encoder Position"=0} ("input cluster"), "Logical Position"=w657, "Encoder Position"=w656) -> (w654:T25)
            "Axis 2" <- w654
            n194 = Unbundle By Name(w675) -> ("register values"=→"register values":i16[])
            n195 = call <vilib>:"Read Encoder Position.vi"("error in (no error)"=w668, "Axis Select"=Axis_Select."Axis 3", "GECO Motion in"=w669) -> ("error out"=w676:errorcluster, "GECO Motion out"=w672:refnum<class "GECO Motion.lvclass">, "Encoder Position"=w658:i32, "Logical Position"=w659:i32)  [unwired: 4 in, 1 out]
            n196 = Bundle(cluster=T25 {"Logical Position"=0, "Encoder Position"=0} ("input cluster"), "Logical Position"=w659, "Encoder Position"=w658) -> (w653:T25)
            "Axis 3" <- w653
            n197 = Bundle By Name(cluster=w675, "GECO Motion out"=w672, "Axis 1 Position"=w655, "Axis 2 Position"=w654, "Axis 3 Position"=w653) -> (w673:T12)
          }
          frame "CloseBoard" {
            w679 = T13[] [enum."Axis 1", enum."Axis 2", enum."Axis 3", enum."Axis 4"] items=["Axis 1", "Axis 2", "Axis 3", "Axis 4"]
            n198 = Unbundle By Name(w687) -> ("GECO_Driver out"=w681:refnum<class "GECO_Driver.lvclass">, "GECO Motion out"=w680:refnum<class "GECO Motion.lvclass">)
            n199 = Flush Queue(queue=w685, error in (no error)=w684) -> (error out=w683:errorcluster)  [unwired: 2 out]
            n200 = for {
              tunnel: [w692] -> w682
              tunnel: w680 -> [w691]
              tunnel: w683 -> [w690]
              tunnel: w679 -> [w688] mode=indexing
              n201 = call <vilib>:"Servo On.vi"("error in (no error)"=w690, "Servo On"=FALSE, "Axis Select"=w688, "GECO Motion in"=w691) -> ("error out"=w695:errorcluster, "Axis Select out"=w694:T13, "GECO Motion out"=w693:refnum<class "GECO Motion.lvclass">)  [unwired: 5 in]
              n202 = call <vilib>:"Single Axis Move Stop.vi"("error in (no error)"=w695, "Axis Select"=w694, "GECO Motion in"=w693) -> ("error out"=w692:errorcluster)  [unwired: 6 in, 2 out]
            }
            n203 = call <vilib>:"Close.vi"("error in (no error)"=w682, "GECO_Driver in"=w681) -> ("error out"=w686:errorcluster)  [unwired: 9 in]
          }
        }
        n204 = Unbundle By Name(w33) -> ("status"=w32:bool)
      }
      frame Error {
      }
    }
    n205 = Tick Count (ms)() -> (millisecond timer value=w22:u32)
    n206 = Subtract(x=w22, y=w21) -> (x-y=→"Program Period":u32)
  }
  n207 = Enqueue Element(queue=w5, element=T19 {"CMD"="Idle", "DATA"=variant}, error in (no error)=w8) -> (error out=w7:errorcluster)  [unwired: 1 in, 2 out]
  n208 = shared-variable ".\\RT_Variables.lvlib\\GyroProgramQueue"() -> (w2:refnum<queue>)  [unwired: 1 in, 1 out]
  n209 = while {
    tunnel: w2 -> [w705]
    tunnel: w3 -> [w704]
    shift-right: [w698] -> _
    shift-left: T20 {"Byte bits"=0, "baud rate"=0, "實際角度"={"A"=0.0, "B"=0.0}, "COM Port"="", "Save Path"=refnum} -> [w699]
    stop <- w700 stop-if-true
    # "Gyro"
    n210 = Dequeue Element(queue=w705, error in (no error)=w704) -> (queue out=w702:refnum<queue>, element=w701:T19, error out=w703:errorcluster)  [unwired: 1 in, 1 out]
    n211 = case shown="No Error" w703 {
      selector: w703 -> [w709 _]
      tunnel: w702 -> [w708 _]
      tunnel: w701 -> [w713 _]
      tunnel: [w706 TRUE] -> w700
      tunnel: w699 -> [w711 w749]
      tunnel: [w710 w749] -> w698
      frame No Error {
        n212 = Unbundle(w713) -> ("CMD"=w712:string)  [unwired: 1 out]
        n213 = case shown="\"Idle\"" w712 {
          tunnel: [w715 w721 w723 w737 w742 w744] -> w710
          tunnel: w711 -> [w715 w722 w723 w737 w742 w744]
          tunnel: w709 -> [w714 w717 _ _ w741 w748]
          tunnel: [w714 w717 w726 w733 w741 w745] -> w707
          tunnel: w708 -> [_ _ w724 w736 _ w746]
          frame Default {
          }
          frame "Idle" {
            # "圖表歸零"
            n214 = property on="實際角度Chart" class="WFChart (strict)"("History Data"=cluster{"X":dbl, "Y":dbl}[] []) -> ()  [unwired: 2 in, 2 out]
            n215 = Bundle By Name(cluster=w722, "COM Port"="Serial Port", "baud rate"="baud rate", "Byte bits"="Byte bits") -> (w721:T20)
          }
          frame "GyroLink" {
            n216 = Enqueue Element(queue=w724, element=T19 {"CMD"="GyroBoardAccess", "DATA"=variant}) -> (error out=w726:errorcluster)  [unwired: 2 in, 2 out]
          }
          frame "GyroBoardAccess" {
            n217 = Unbundle By Name(w737) -> ("COM Port"=w730:refnum<visa-resource-name>)
            n218 = call-poly "VISA Configure Serial Port"("VISA resource name"=w730, "baud rate (9600)"=u32 115200, "data bits (8)"=u16 8) -> ("VISA resource name out"=w728:refnum<visa-resource-name>, "error out"=w727:errorcluster)  [unwired: 11 in]
            n219 = VISA Read(VISA resource name=w728, byte count=u32 13, error in (no error)=w727) -> (read buffer=w740:string, error out=w739:errorcluster)  [unwired: 2 out]
            n220 = call "Arduino角度.vi"("error in"=w739, "read buffer"=w740) -> ("error out"=w734:errorcluster, "Waveform Chart"=→"實際角度" →"實際角度Chart":cluster{dbl, dbl})  [unwired: 2 in]
            n221 = Enqueue Element(queue=w736, element=T19 {"CMD"="GyroBoardAccess", "DATA"=variant}, error in (no error)=w734) -> (error out=w733:errorcluster)  [unwired: 1 in, 2 out]
          }
          frame "GyroPanelUpdate" {
            n222 = Unbundle By Name(w742) -> ()  [unwired: 1 out]
          }
          frame "CloseBoard" {
            n223 = Unbundle By Name(w744) -> ("COM Port"=w743:refnum<visa-resource-name>)
            n224 = Flush Queue(queue=w746, error in (no error)=w748) -> (error out=w747:errorcluster)  [unwired: 2 out]
            n225 = VISA Close(VISA resource name=w743, error in (no error)=w747) -> (error out=w745:errorcluster)
          }
        }
        n226 = Unbundle By Name(w707) -> ("status"=w706:bool)
      }
      frame Error {
      }
    }
  }
  n227 = while {
    shift-right: [w753] -> w20
    shift-left: w7 -> [w756]
    tunnel: w6 -> [w757]
    tunnel: w5 -> [w751]
    stop <- w754 stop-if-true
    # "EventLoop"
    n228 = event shown="[3] \"Connect\": Value Change" {
      selector: _ -> [_ _ _ _ _ _ _ _ _ _ _ _]
      dyn-events: _ -> [_ _ _ _ _ _ _ _ _ _ _ _]
      timeout: _ -> [_ _ _ _ _ _ _ _ _ _ _ _]
      tunnel: w757 -> [w761 w765 w769 w776 w780 w784 w790 w794 _ _ w812 _]
      tunnel: w756 -> [w760 w764 w768 w775 w779 w783 w789 w793 w800 w806 w811 w814]
      tunnel: [w759 w763 w767 w772 w778 w782 w788 w792 w799 w805 w809 w814] -> w753
      tunnel: [_ _ _ _ _ _ _ _ _ _ _ w813] -> w755
      tunnel: w751 -> [_ _ _ w770 _ _ _ _ w797 w803 w807 _]
      event "Modbus Number of Inputs", "Serial Port", "TCP slave port", "baud rate", "Byte bits", "Modbus Address Starting": Value Change {
        n229 = event-data() -> ()  [unwired: 1 in, 1 out]
        n230 = Enqueue Element(queue=w761, element=T19 {"CMD"="SettingChange", "DATA"=variant}, error in (no error)=w760) -> (error out=w759:errorcluster)  [unwired: 1 in, 2 out]
      }
      event "Forward Enable?", "Reverse Enable?", "Motion Operation Mode", "Target Position (0)", "Acceleration (100000)", "Velocity (10000)", "Deacceleration (100000)", "Servo on": Value Change {
        n231 = event-data() -> ()  [unwired: 1 in, 1 out]
        n232 = Enqueue Element(queue=w765, element=T19 {"CMD"="ServoSetting", "DATA"=variant}, error in (no error)=w764) -> (error out=w763:errorcluster)  [unwired: 1 in, 2 out]
      }
      event "Z", "A", "B", "PID gains", "PID gains 2", "PID gains 3": Value Change {
        n233 = event-data() -> ()  [unwired: 1 in, 2 out]
        n234 = Enqueue Element(queue=w769, element=T19 {"CMD"="PIDSetting", "DATA"=variant}, error in (no error)=w768) -> (error out=w767:errorcluster)  [unwired: 1 in, 2 out]
      }
      event "Connect": Value Change {
        n235 = event-data() -> ()  [unwired: 1 in, 1 out]
        n236 = Enqueue Element(queue=w776, element=T19 {"CMD"="LinkBoard", "DATA"=variant}, error in (no error)=w775) -> (error out=w773:errorcluster)  [unwired: 1 in, 2 out]
        n237 = Enqueue Element(queue=w770, element=T19 {"CMD"="GyroLink", "DATA"=variant}, error in (no error)=w773) -> (error out=w772:errorcluster)  [unwired: 1 in, 2 out]
      }
      event "ServoButtonControl.AlarmReset": Value Change {
        n238 = event-data() -> ()  [unwired: 1 in, 1 out]
        n239 = Enqueue Element(queue=w780, element=T19 {"CMD"="AlarmReset", "DATA"=variant}, error in (no error)=w779) -> (error out=w778:errorcluster)  [unwired: 1 in, 2 out]
      }
      event "ServoButtonControl.Reset Encoder Position": Value Change {
        n240 = event-data() -> ()  [unwired: 1 in, 1 out]
        n241 = Enqueue Element(queue=w784, element=T19 {"CMD"="EncoderReset", "DATA"=variant}, error in (no error)=w783) -> (error out=w782:errorcluster)  [unwired: 1 in, 2 out]
      }
      event "ServoButtonControl": Value Change {
        n242 = event-data() -> ()  [unwired: 1 in, 1 out]
        n243 = Bundle By Name(cluster=T19 {"CMD"="Shooting", "DATA"=variant} ("element"), "DATA"="ServoButtonControl") -> (w786:T19)
        n244 = Enqueue Element(queue=w790, element=w786, error in (no error)=w789) -> (error out=w788:errorcluster)  [unwired: 1 in, 2 out]
      }
      event "ZABStop", "ZAB Start": Value Change {
        n245 = event-data() -> ()  [unwired: 1 in, 2 out]
        n246 = Enqueue Element(queue=w794, element=T19 {"CMD"="ZABMove", "DATA"=variant}, error in (no error)=w793) -> (error out=w792:errorcluster)  [unwired: 1 in, 2 out]
      }
      event "TimerON": Value Change {
        n247 = event-data() -> ("NewVal"=w795:bool)  [unwired: 1 in]
        n248 = Bundle By Name(cluster=T19 {"CMD"="ChangeTimerState", "DATA"=variant} ("element"), "DATA"=w795) -> (w796:T19)
        n249 = Enqueue Element(queue=w797, element=w796, error in (no error)=w800) -> (error out=w799:errorcluster)  [unwired: 1 in, 2 out]
      }
      event "Timer(ms)": Value Change {
        n250 = event-data() -> ("NewVal"=w801:i32)  [unwired: 1 in]
        n251 = Bundle By Name(cluster=T19 {"CMD"="ChangeTimerCount", "DATA"=variant} ("element"), "DATA"=w801) -> (w802:T19)
        n252 = Enqueue Element(queue=w803, element=w802, error in (no error)=w806) -> (error out=w805:errorcluster)  [unwired: 1 in, 2 out]
      }
      event "Close": Value Change {
        w808 = T19 {"CMD"="CloseBoard", "DATA"=variant} ("element")
        n253 = event-data() -> ()  [unwired: 1 in, 1 out]
        n254 = Enqueue Element At Opposite End(queue=w812, element=w808, error in (no error)=w811) -> (error out=w810:errorcluster)  [unwired: 1 in, 2 out]
        n255 = Enqueue Element At Opposite End(queue=w807, element=w808, error in (no error)=w810) -> (error out=w809:errorcluster)  [unwired: 1 in, 2 out]
      }
      event Panel Close? {
        w813 = TRUE
        n256 = event-data() -> ()  [unwired: 1 in, 1 out]
        n257 = event-data("Discard?"=w813) -> ()  [unwired: 1 in, 1 out]
      }
    }
    n258 = Unbundle By Name(w753) -> ("status"=w752:bool)
    n259 = Or(x=w752, y=w755) -> (x .or. y?=w754:bool)
  }
  n260 = Release Queue(queue=w5, error in (no error)=w20) -> (error out=w10:errorcluster)  [unwired: 1 in, 2 out]
  n261 = Release Queue(queue=w6, error in (no error)=w10) -> ()  [unwired: 1 in, 3 out]
